vi "Main.vi"() -> ()   [LabVIEW 2016]
doc: "Use this template to create an application that executes until you click the Stop button. Unlike the Single Loop Application VI that uses polling, this VI uses the Event Structure."
uses:
  <vilib>/userdefined/High Color/IMAQdx.ctl
  <vilib>/Utility/file.llb/Write To Spreadsheet File (string).vi
  <vilib>/Utility/file.llb/Read From Spreadsheet File (string).vi
  Library_alfa.lvlib
  <vilib>/vision/driver/NI_Vision_Acquisition_Software.lvlib
  <vilib>/vision/NI_Vision_Development_Module.lvlib
panel:
  out "индикация видео":T1(plugin-control)
  in  "Media Stop Button":bool
  in  "Play Button":bool
  in  "Камера":T2
  in  "Область измерения":T3 {"Rotation" format="%.2f"; "Left" scale=0.0..1024.0; "Right" scale=0.0..1280.0}
  in  "Параметры измерения":T4={"Contrast"=40, "Filter width"=4, "Steepness"=2, "Subsampling Ratio"=5, "Show Search Area"=FALSE, "Show Search Lines"=FALSE, "Show Edges Found"=FALSE, "Show Result"=TRUE}
  in  "Рабочий цвет":u32(colorbox)
  in  "Калибровка":u32(colorbox)
  in  "Задержка":u32
  in  "Уровень бинаризации":T5={"Нижний предел"=128.0, "Верхний предел"=255.0} {"Верхний предел" format="%.2f"; "Нижний предел" format="%.2f"}
  in  "Фильтр":i32(ring)=1 items=["Red", "Green", "Blue", "Hue", "Saturation", "Luminance", "Value", "Intensity"]
  out "Индикатор камеры":bool
  in  "Blank Button":bool
  out "Индикатор камеры 2":bool
  in  "Сохранить настройки":bool
  in  "Tab Control 3":enum32{"Настройки видео", "Регулятор"}(tab)
  in  "автоматическое включение регулятора":bool caption="Автоматическое включение регулятора"
  out "Индикатор автозапуска регулятора":bool
  out "Максимальная подача (мм/мин)2":string caption="Max скорость\n(mm/min)"
  out "Boolean":bool
  in  "Регулятор":bool
  out "текущая скорость\n(mm/min)":string
  out "текущее значение\nзазора (mm)":string
  out "Задание \nзазора (mm)":string
  in  "взять зазор":bool caption="Регулятор"
  out "Марка сплава":string
  in  "Положение толкателя (mm)":dbl(slide) scale=0.0..100.0
  in  "ND HEAT BUT":bool
  in  "ND HEAT LED":bool
  out "PT 4txt":string caption="Вакуум в камере\nPT2 (torr)"
  out "PT4 2":u16(ring)
  out "NL2":u16(ring)
  in  "V5014":dbl
  out "давление 2":bool
  out "давление 1":bool
  in  "V5012_SP_He_PC2":dbl
  out "Air":bool
  in  "ПЛАЗМАТРОН В ИСХОДНОЕ":bool
  in  "Продол назад":bool
  in  "V5011_SP_He_PC2":dbl
  in  "V5010_SP_C1":dbl
  out "PT 4":string caption="Вакуум в камере\nPT2 (torr)"
  in  "PT4":dbl
  in  "M_PLasmatron":dbl
  out "V барабаны 2":dbl
  in  "Tab Control 2":enum32{"X1", "X2", "Y"}(tab)
  out "X240":bool[](array[boolean])
  out "ОП1 Х1 5":string[](array[string])
  out "X200":bool[](array[boolean])
  out "ОП1 Х1 4":string[](array[string])
  out "X140":bool[](array[boolean])
  out "ОП1 Х1 3":string[](array[string])
  out "X100":bool[](array[boolean])
  out "ОП1 Х1 2":string[](array[string])
  out "X400":bool[](array[boolean])
  out "ОП1 Х1 8":string[](array[string])
  out "X340":bool[](array[boolean])
  out "ОП1 Х1 7":string[](array[string])
  out "X300":bool[](array[boolean])
  out "ОП1 Х1 6":string[](array[string])
  out "Y120":bool[](array[boolean])
  out "ОП1 Х1 10":string[](array[string])
  out "Y60":bool[](array[boolean])
  out "ОП1 Х1 9":string[](array[string])
  out "Air 4":bool
  in  "PT3 2":dbl
  out "V вращ. бараб 2":string caption="V заготовки"
  out "LONGITUDINAL SPEED":string
  out "PLASMATRON SPEED":string
  in  "mac3":bool
  in  "Ошибка 2":i16 format="%x"
  in  "Скорость пп 2":i16
  out "Полож заг сер":bool
  out "Полож заг нач":bool caption="НАЧАЛО"
  out "Полож заг кон":bool
  out "Полож плазм кон":bool caption="Конец"
  out "Полож плазм сер":bool caption="Пром."
  out "Полож плазм  нач":bool caption="Начало"
  in  "МАКСИМАЛЬНАЯ СКОРОСТЬ ПП К":bool
  in  "v4066_cкорость подачи плазматрона":dbl
  in  "v4065_cкорость подачи":dbl
  in  "V7045_I_ist":dbl
  in  "V7045_U_ist":dbl
  in  "Действующий ток на плазматроне":string caption="Ток А"
  out "V заготовки":string
  in  "D, заготовки":i16
  in  "Закончить автораспыление":bool
  in  "Автораспыление доплавить":bool
  in  "Автораспыление начать":bool
  in  "задание тока А":string caption="Задание, А"
  in  "ПОДАЧА ЗАГОТОВКИ":bool
  in  "stop 2":bool
  in  "SP_зазор":dbl
  in  "PV_зазор":dbl
  in  "max out":dbl
  in  "out":dbl
  out "Distance зазор":sgl format="%.2f"
  out "x/y":dbl
  out "x*y":dbl
  out "16bit integer":i16
  in  "Numeric":i16
  in  "Т6":dbl
  in  "Улавливатель закрыть":bool
  in  "Улавливатель открыть":bool
  in  "Ролик прижать":bool
  in  "Ролик отжать":bool
  in  "PE3":dbl
  in  "PE2":dbl
  in  "PE1":dbl
  in  "ЗАДАНИЕ ТОКА":i16
  in  "ГС - Закрыть":bool
  in  "ГС -Открыть":bool
  out "ГС - Плазматрон":string caption="Плазматрон"
  out "ГС - Камера":string caption="Камера"
  in  "Скорость пп":i16
  in  "V барабаны задание":dbl
  in  "Выход":bool
  in  "ГС ПТ":i16
  in  "ГС камера":i16
  in  "V барабаны":dbl
  in  "Т5":dbl
  in  "Т4":dbl
  in  "Т3":dbl
  in  "Т2":dbl
  in  "Т1":dbl
  in  "Ошибка":i16
  in  "PT3":dbl
  in  "PT2":dbl
  in  "PT1":dbl
  in  "y120":i32
  in  "y60":i32
  in  "x400":i32
  in  "x340":i32
  in  "x300":i32
  in  "x240":i32
  in  "x200":i32
  in  "x140":i32
  in  "x100":i32
  in  "Tab Control":enum32{"Вакуум", "Распыление", "Осциллограмма"}(tab)
  in  "откачка стоп 2":bool
  out "Распыление":bool
  out "Вакуум":bool
  out "Газ":bool
  out "VP4":u16(ring)
  out "PD2":u16(ring)
  out "VP2":u16(ring)
  in  "Slide":dbl(slide) scale=0.0..99.0
  out "EV1":u16(ring)
  out "EV2":u16(ring)
  out "EV3.3":u16(ring)
  out "EV3.2":u16(ring)
  out "PE2":u16(ring)
  out "PE2":string caption="Вакуум в камере\nPT2 (torr)"
  out "CO1":u16(ring)
  out "CO2":u16(ring)
  out "EV3.1":u16(ring)
  out "CO3":u16(ring)
  out "P1":u16(ring)
  out "PE1":u16(ring)
  out "PE1":string caption="Вакуум в камере\nPT2 (torr)"
  out "PE3":u16(ring)
  out "PE3":string caption="Вакуум в камере\nPT2 (torr)"
  out "VP1":u16(ring)
  out "PT3":u16(ring)
  out "PT2":u16(ring)
  out "PT 2":string caption="Вакуум в камере\nPT2 (torr)"
  out "VP3":u16(ring)
  out "VP5":u16(ring)
  out "PD1":u16(ring)
  out "PT1":u16(ring)
  out "PT 1":string caption="Вакуум в камере\nPT2 (torr)"
  out "NZ1":u16(ring)
  out "NR1":u16(ring)
  out "NL1":u16(ring)
  out "PT 3":string caption="Вакуум в камере\nPT2 (torr)"
  out "SP Presure Ar PC2":string caption="SP C1 (kgf/cm^2)"
  in  "напустить аргон в ресивер":bool
  in  "mac6":bool
  out "SP Presure He PC2":string caption="SP C1 (kgf/cm^2)"
  in  "mac5":bool
  in  "напустить гелий в ресивер":bool
  out "SP Presure C1":string caption="SP C1 (kgf/cm^2)"
  in  "mac 4":bool
  in  "напустить газ в камеру":bool
  in  "forvacuum":bool
  in  "forvakuum led":bool
  in  "откачка стоп":bool
  in  "откачка стоп индик":bool
  in  "откачать рабочий вакуум":bool
  in  "mac 2":bool
  out "ИНдикатор положения полки":string
  in  "ЗУ-вверх":bool
  in  "Пауза допыления":string caption="Пауза допыления (sec)"
  out "C212":bool
  out "УГ_закрыт":bool caption="Отжат"
  out "УГ_открыт":bool caption="Прижат"
  out "ролик_отжат":bool caption="Вверху"
  out "ролик_прижат":bool caption="Внизу"
  out "max Speed":string caption="Максимальная \nСкорость (r/min)"
  out "ТЕМП КАМЕРА":string caption="T газ (C°)"
  in  "Скорость ПП 2":string caption="Скорость плазматрона\n(mm/min)"
  in  "Скорость ПП":string caption="Скорость толкателя (mm/min)"
  out "ТЕМП РОЛИК":string caption="T ролик (C°)"
  out "ПОДШ. 2.2":string caption="T4 (C°)"
  out "ПОДШ. 2.1":string caption="T3 (C°)"
  out "ПОДШ. 1.2":string caption="T2 (C°)"
  out "ПОДШ. 1.1":string caption="T1 (C°)"
  out "P плазматрон (bar)":string
  out "P камера (bar)":string
  out "I_ist":string caption="Ток (A)"
  out "U_ist":string caption="Напряжение (V)"
  out "Диаметр заг.":string caption="Диаметр (mm)"
  out "V задания":string caption="Скорость вращения (r/min)"
  out "V вращ. бараб":string caption="Частота вращения (r/min)"
  in  "ПЛАЗМАТРОН В ИСХОДНОЕ 2":bool
  out "Частота вращения":dbl(graph)
  out "Значение зазора":dbl(graph)
  out "Скорость толкателя":dbl(graph)
  out "Ток":dbl(graph)
  out "Напряжение":dbl(graph)
  out "voto plasmatron":string caption="моточасы работы\nплазматрона"
  out "текущее время":string
  in  "Arhive":bool
  # "Ролик"
  # "Улавливатель ОГ"
  # "PLASMATRON"
  # "Обработка"
  # "БАРАБАНЫ"
  # "РАСПЫЛЕНИЕ ЗАГОТОВКИ"
  # "Температура"
  # "3A3.1 X100-X137"
  # "3A3.2 X140-177"
  # "3A4 X200-X237"
  # "3A5.1 X240-X277"
  # "3A5.2 X300-X337"
  # "3A6 X340-X377"
  # "3A8 X400-X437"
  # "2A8 Y60-Y117"
  # "3A7 Y120-Y157"
  # "Положение толкателя"
  # "Положение плазматрона"
  # "Газовая система"
  # "VF1"
  # "Ar,He"
  # "PC1"
  # "PC2"
  # "Толкатель"
  # "Прижим крышки"
  # "Прижимной ролик"
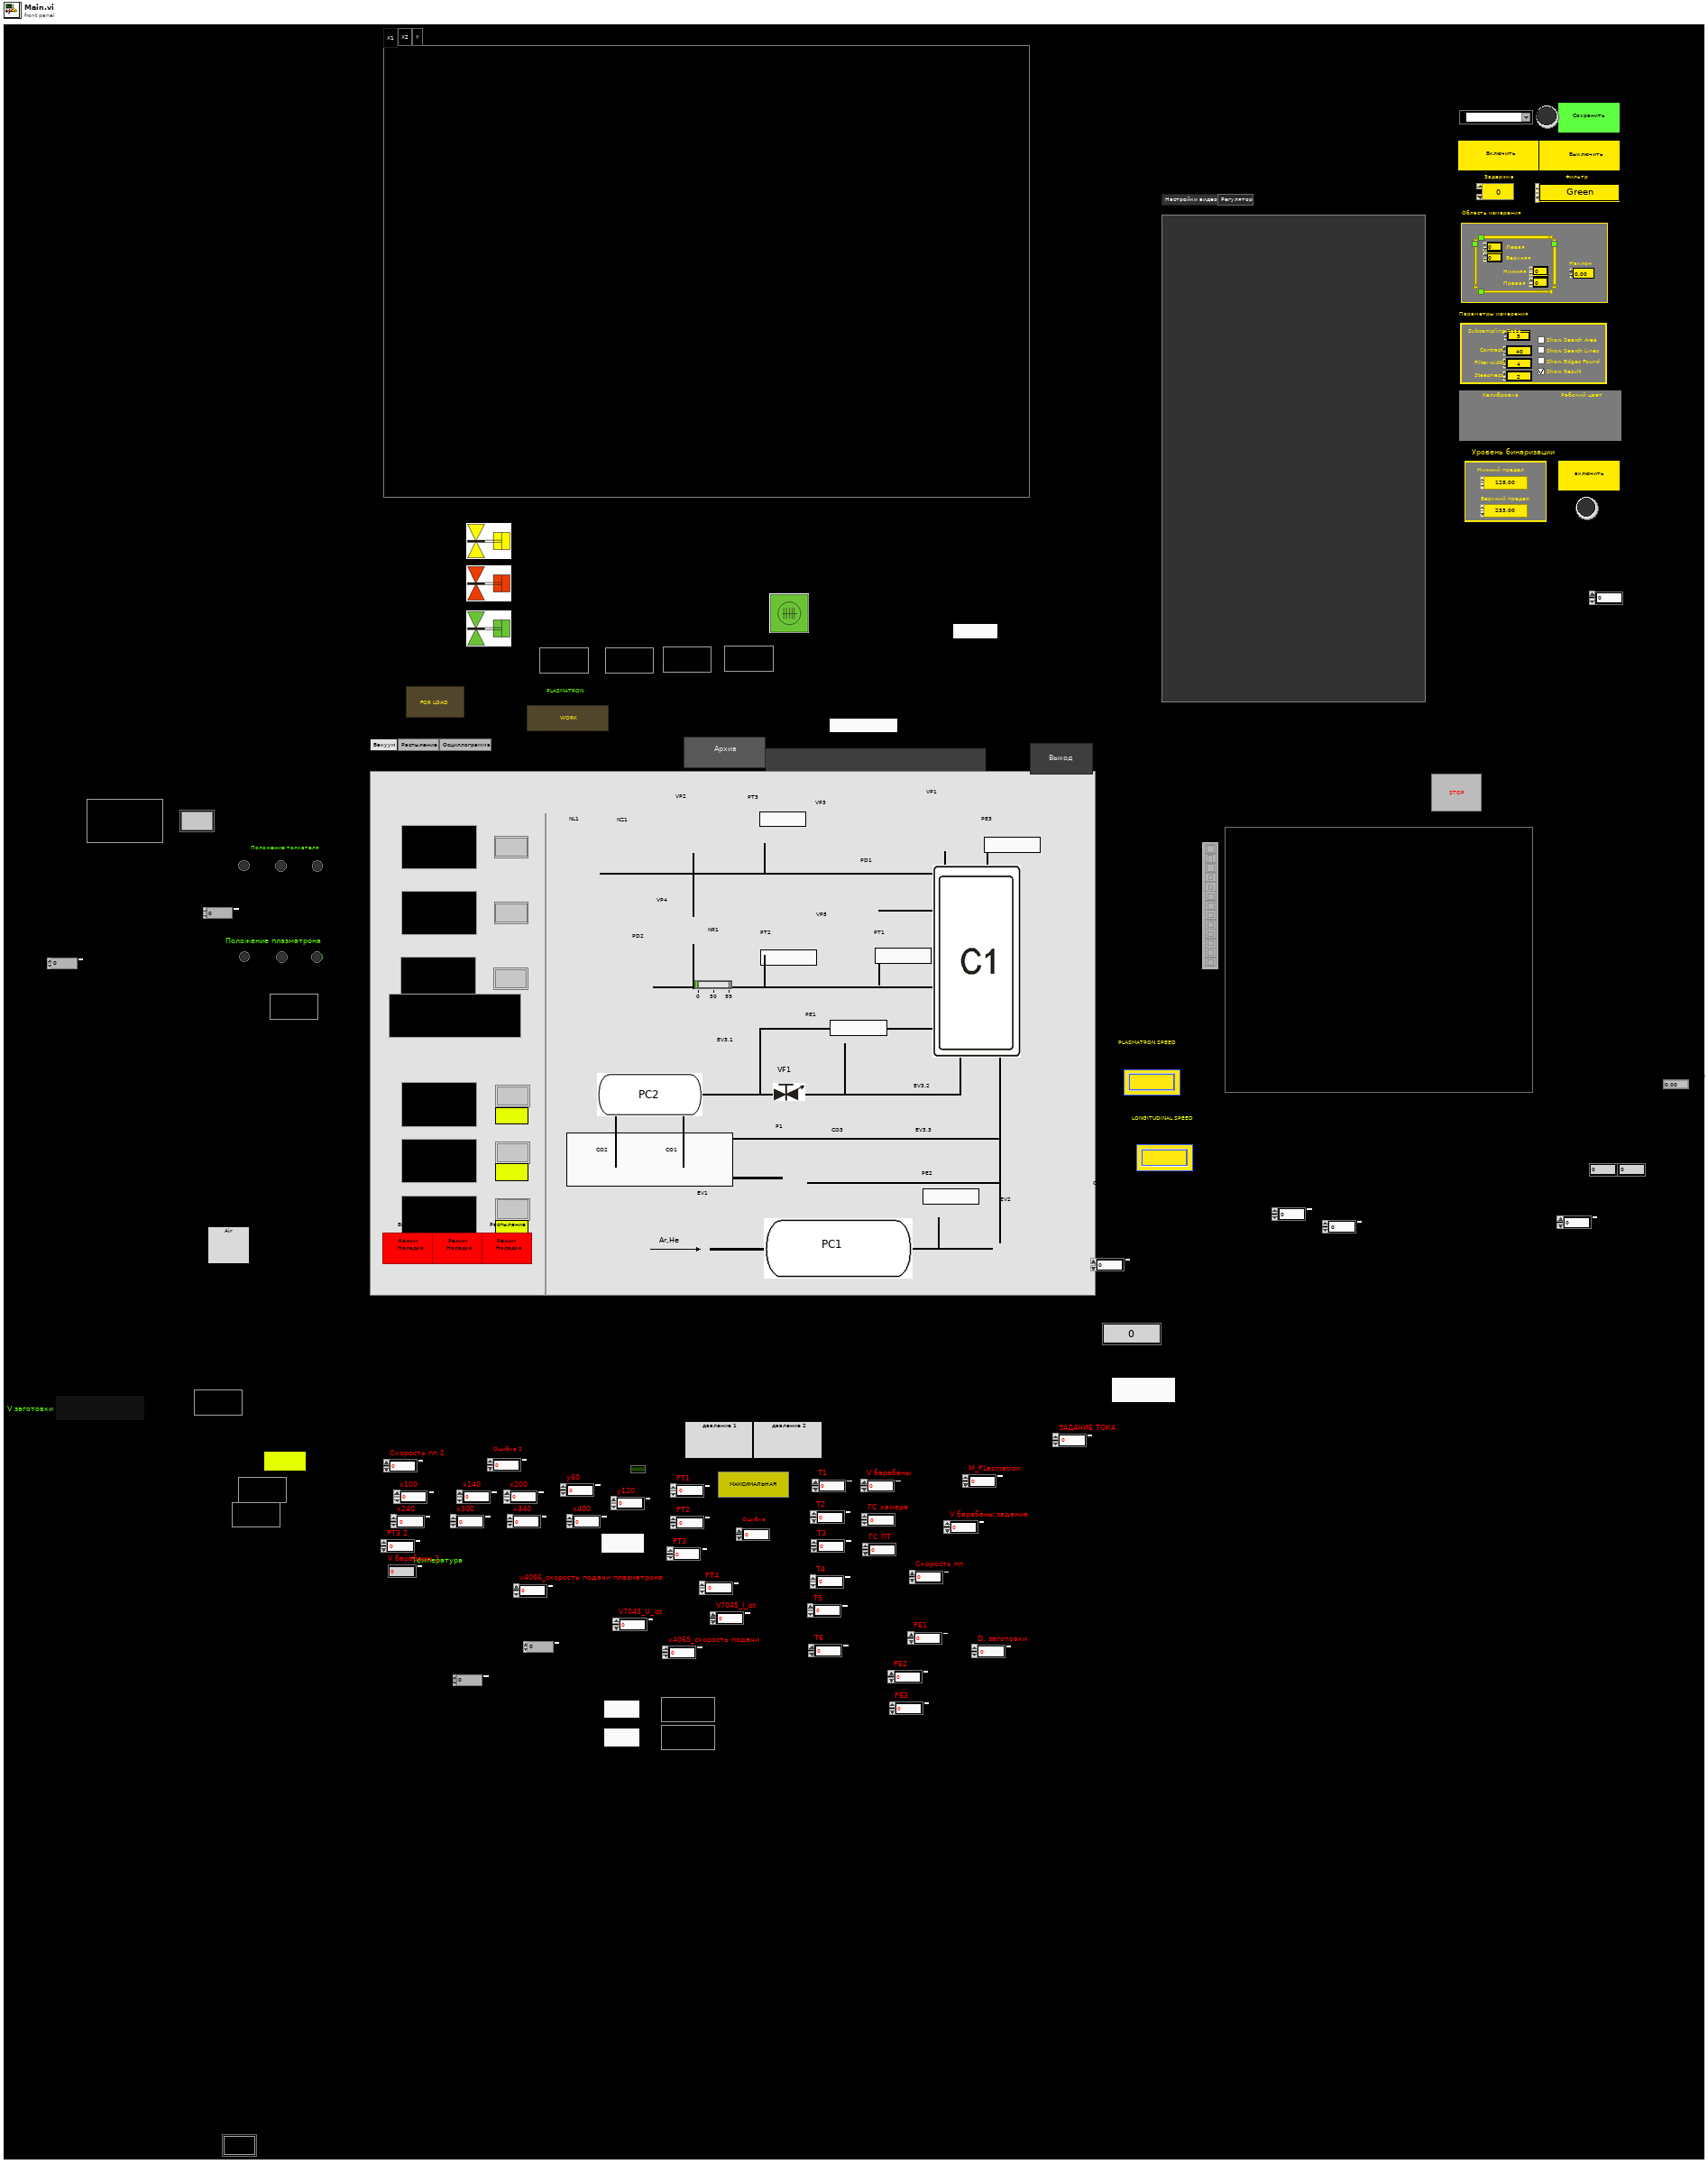
[diagram p1: front panel]
types:
  T1 = typedef "IMAQ Image.ctl" = refnum<image>
  T2 = typedef "Library_alfa.lvlib/IMAQdx.ctl" = refnum<k21>
  T3 = typedef "IMAQ Rectangle" = cluster{"Left":i32, "Top":i32, "Right":i32, "Bottom":i32, "Rotation":dbl}
  T4 = cluster{"Contrast":i32, "Filter width":i32, "Steepness":i32, "Subsampling Ratio":u32, "Show Search Area":bool, "Show Search Lines":bool, "Show Edges Found":bool, "Show Result":bool}
  T5 = cluster{"Нижний предел":sgl, "Верхний предел":sgl}
  T6 = enum16{"open", "replace", "create", "open or create", "replace or create", "replace or create with confirmation"}
  T7 = enum8{"Enabled", "Disabled", "Disabled and Grayed Out"}
  T8 = cluster{i32, i32, i32, u32, "Boolean":bool, "Boolean":bool, "Boolean":bool, "Boolean":bool}
  T9 = typedef "Image Type" = u32
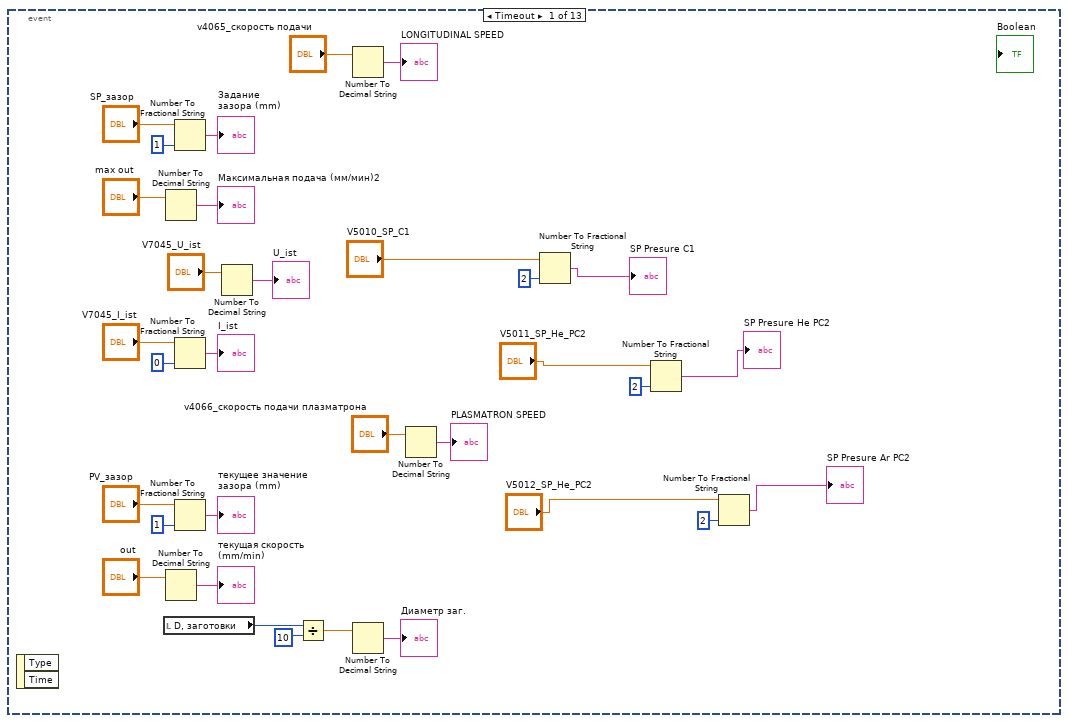
[diagram p6: hidden frame]
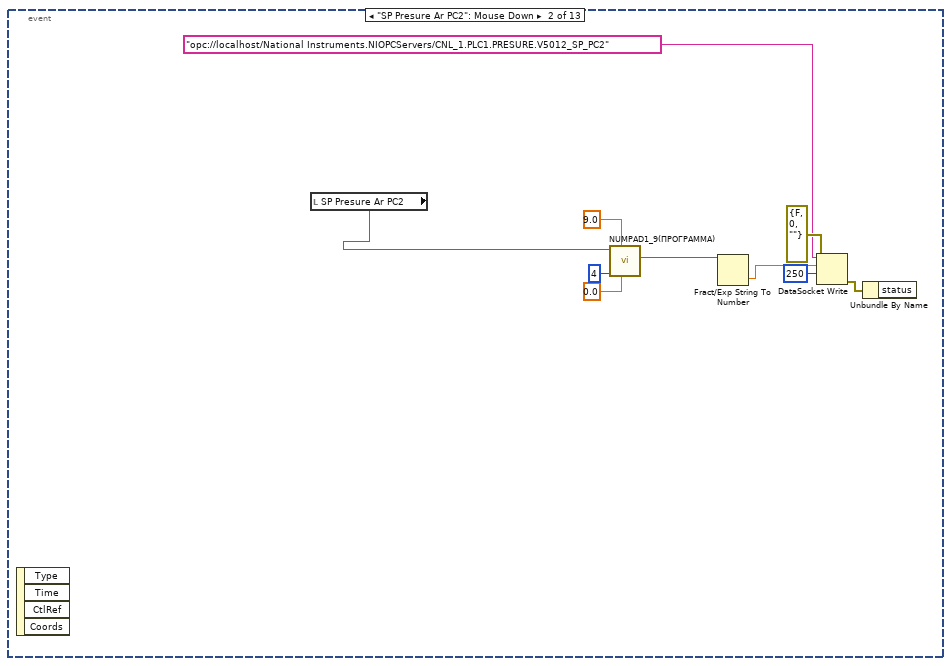
[diagram p7: hidden frame]
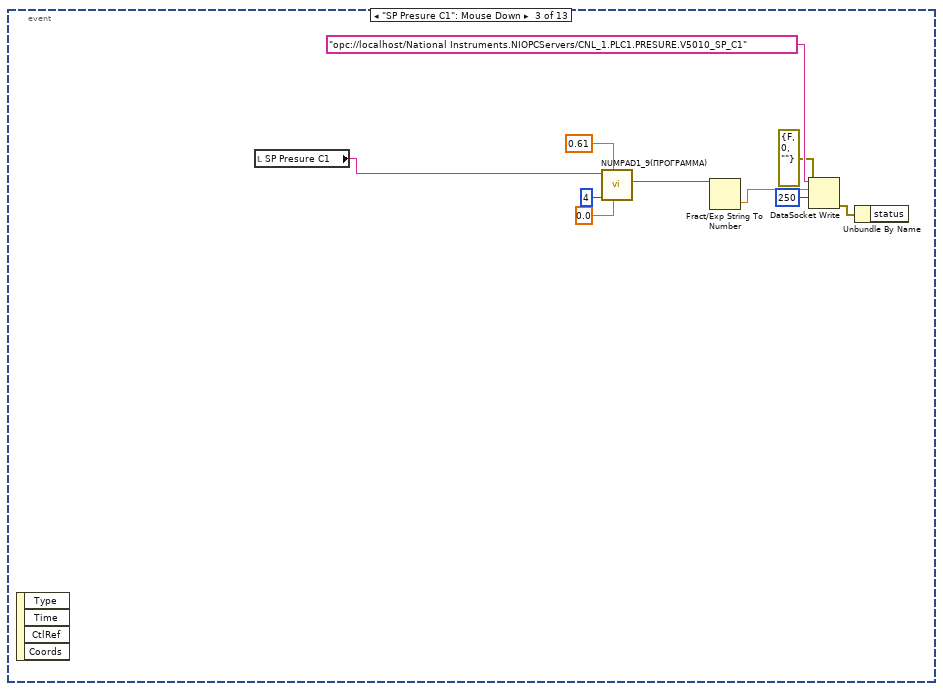
[diagram p8: hidden frame]
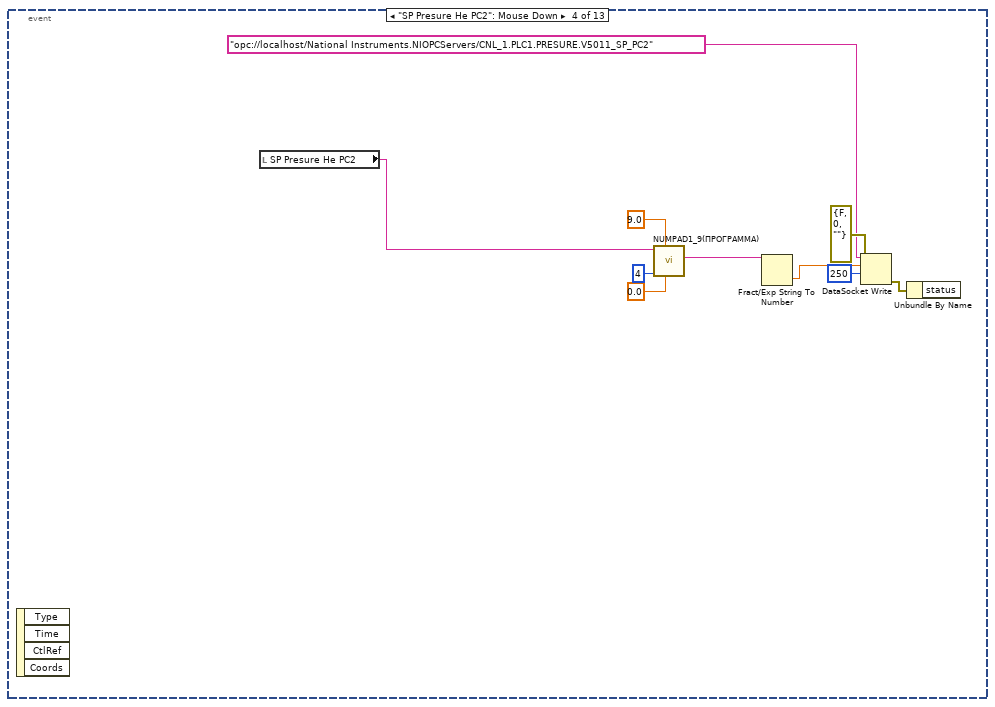
[diagram p9: hidden frame]
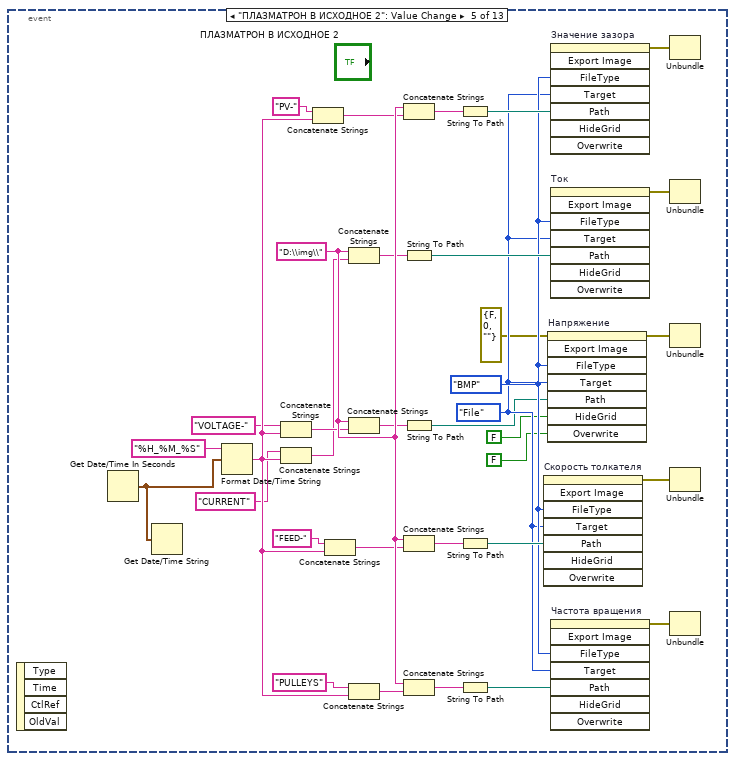
[diagram p10: hidden frame]
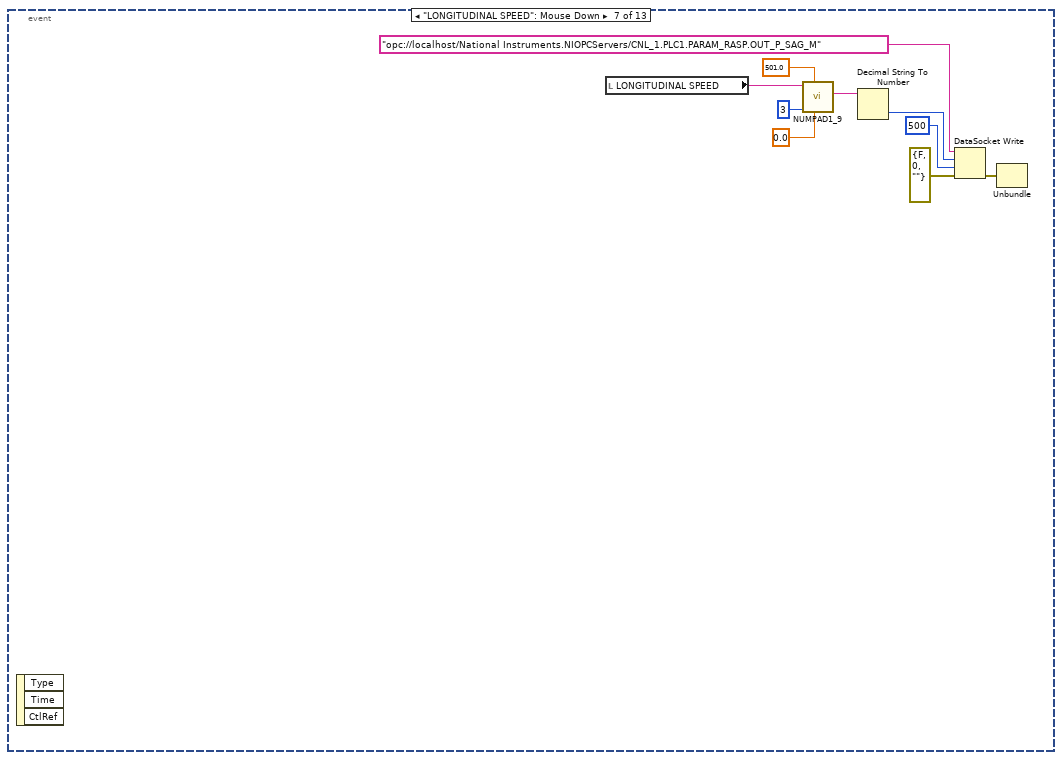
[diagram p11: hidden frame]
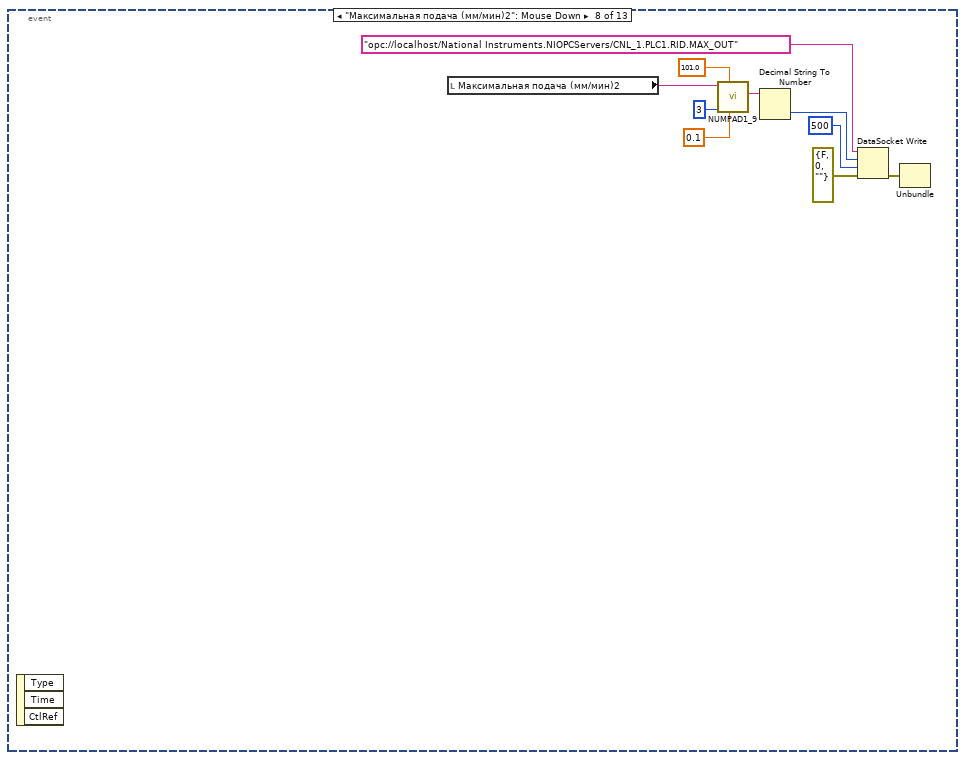
[diagram p12: hidden frame]
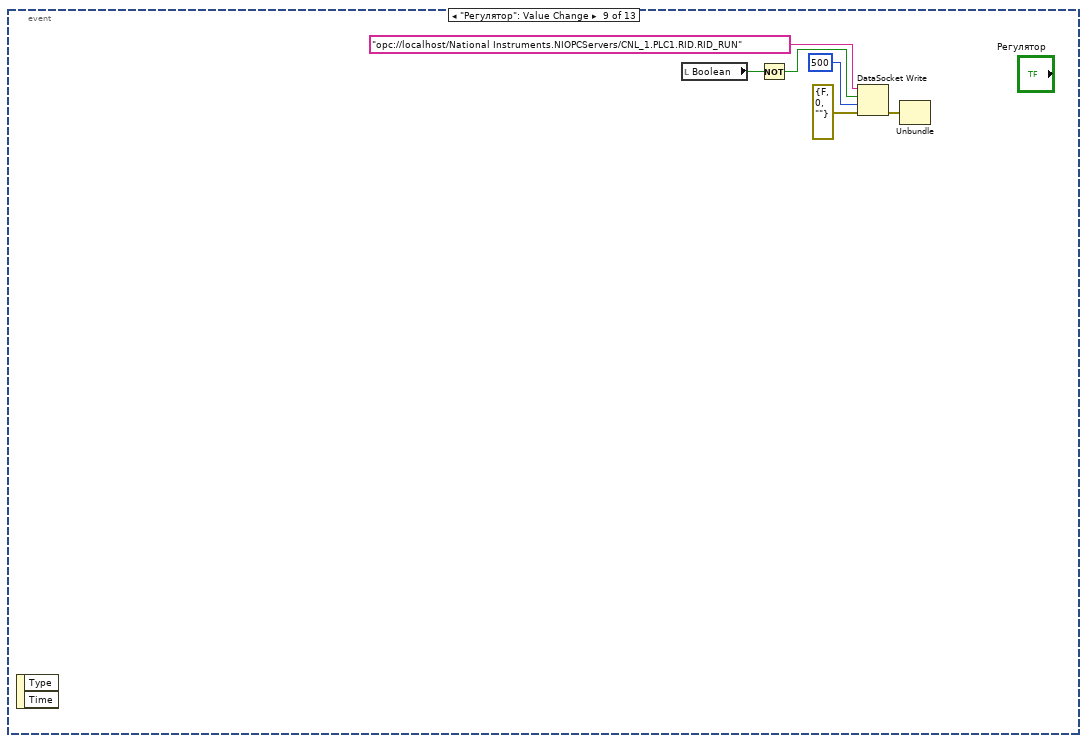
[diagram p13: hidden frame]
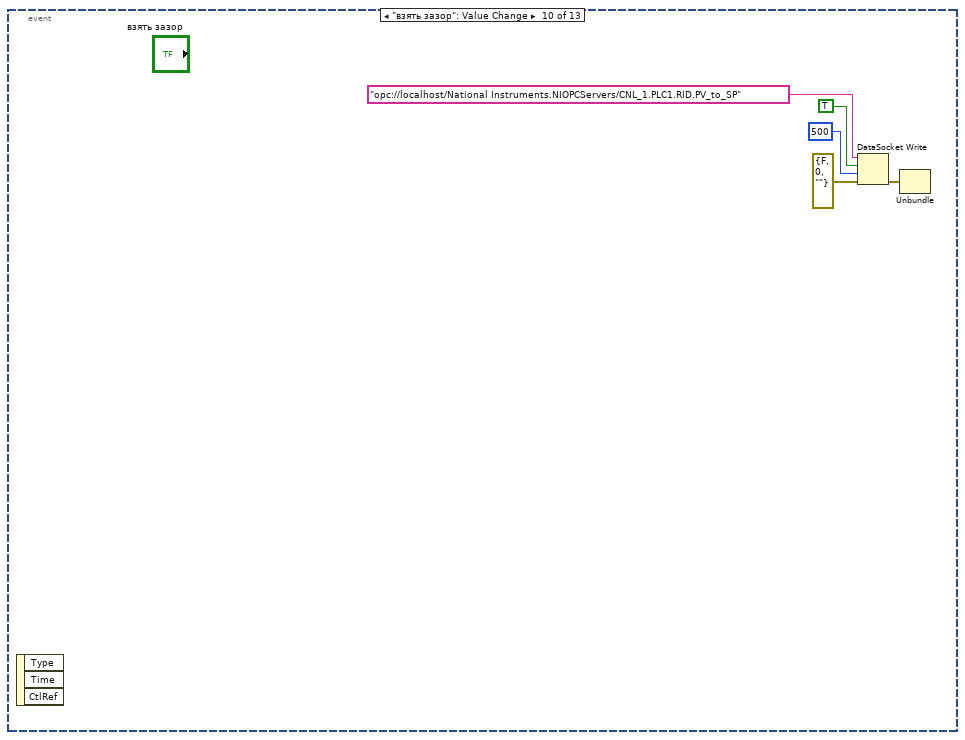
[diagram p14: hidden frame]
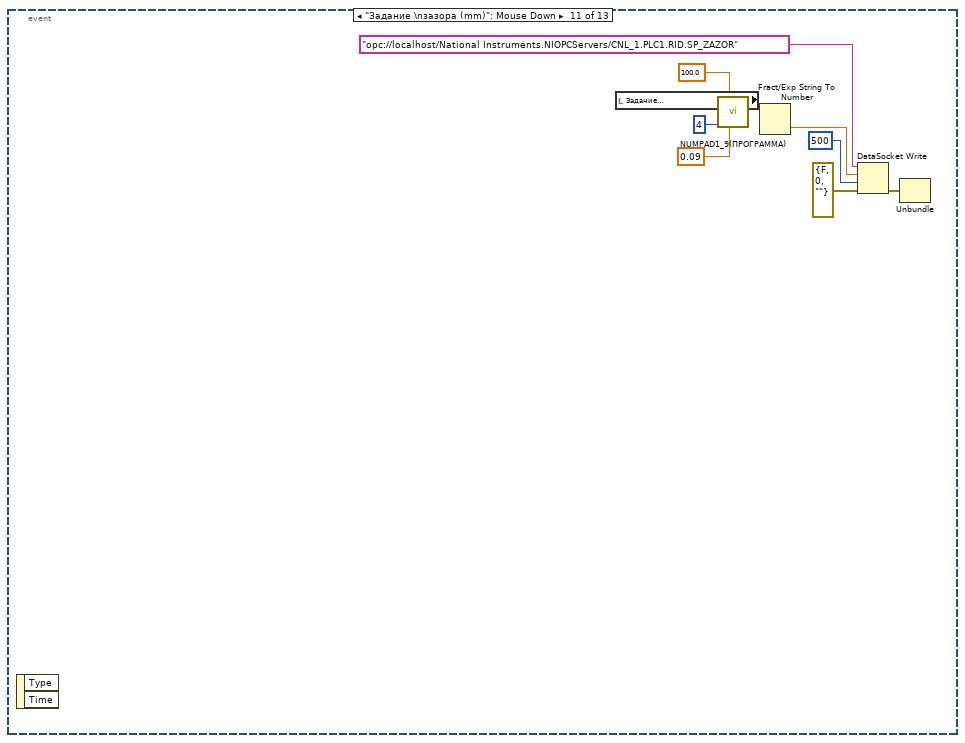
[diagram p15: hidden frame]
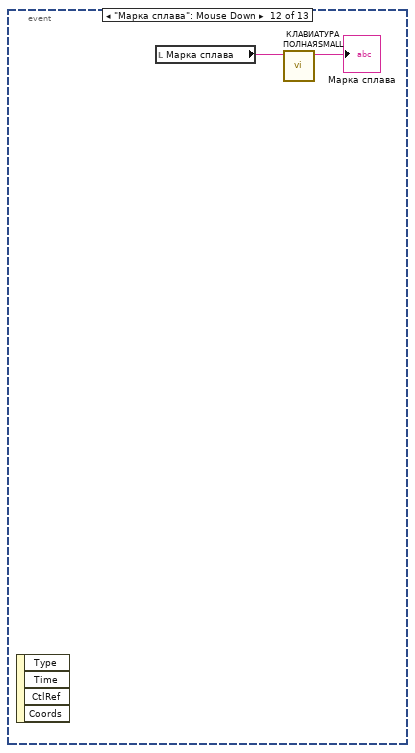
[diagram p16: hidden frame]
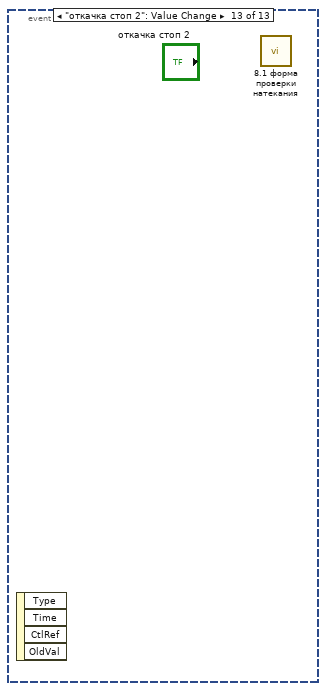
[diagram p17: hidden frame]
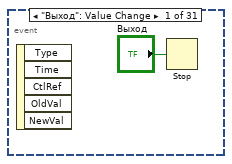
[diagram p19: hidden frame]
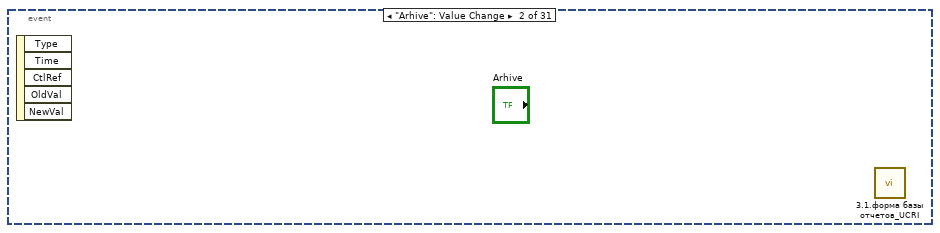
[diagram p20: hidden frame]
diagram:
  n1 = while {
    stop <- "stop 2" stop-if-true
    n2 = Wait Until Next ms Multiple(millisecond multiple=u32 250) -> ()  [unwired: 1 out]
    n3 = event shown="[5] \"PLASMATRON SPEED\": Mouse Down" {
      selector: _ -> [_ _ _ _ _ _ _ _ _ _ _ _ _]
      dyn-events: _ -> [_ _ _ _ _ _ _ _ _ _ _ _ _]
      timeout: 250 -> [_ _ _ _ _ _ _ _ _ _ _ _ _]
      event Timeout {
        n4 = event-data() -> ()  [unwired: 1 in, 2 out]
        n5 = local read "D, заготовки"() -> (w30:i16)
        n6 = Number To Decimal String(number="max out") -> (decimal integer string=→"Максимальная подача (мм/мин)2":string)  [unwired: 1 in]
        n7 = Number To Decimal String(number="out") -> (decimal integer string=→"текущая скорость\n(mm/min)":string)  [unwired: 1 in]
        n8 = Number To Fractional String(number="SP_зазор", precision (6)=i16 1) -> (F-format string=→"Задание \nзазора (mm)":string)  [unwired: 2 in]
        n9 = Number To Fractional String(number="V7045_I_ist", precision (6)=i16 0) -> (F-format string=→"I_ist":string)  [unwired: 2 in]
        n10 = Number To Fractional String(number="PV_зазор", precision (6)=i16 1) -> (F-format string=→"текущее значение\nзазора (mm)":string)  [unwired: 2 in]
        n11 = Number To Decimal String(number="V7045_U_ist") -> (decimal integer string=→"U_ist":string)  [unwired: 1 in]
        n12 = Divide(x=w30, y=i16 10) -> (x/y=w28:dbl)
        n13 = Number To Decimal String(number="v4065_cкорость подачи") -> (decimal integer string=→"LONGITUDINAL SPEED":string)  [unwired: 1 in]
        n14 = Number To Decimal String(number=w28) -> (decimal integer string=→"Диаметр заг.":string)  [unwired: 1 in]
        n15 = Number To Decimal String(number="v4066_cкорость подачи плазматрона") -> (decimal integer string=→"PLASMATRON SPEED":string)  [unwired: 1 in]
        n16 = Number To Fractional String(number="V5010_SP_C1", precision (6)=i16 2) -> (F-format string=→"SP Presure C1":string)  [unwired: 2 in]
        n17 = Number To Fractional String(number="V5011_SP_He_PC2", precision (6)=i16 2) -> (F-format string=→"SP Presure He PC2":string)  [unwired: 2 in]
        n18 = Number To Fractional String(number="V5012_SP_He_PC2", precision (6)=i16 2) -> (F-format string=→"SP Presure Ar PC2":string)  [unwired: 2 in]
      }
      event "SP Presure Ar PC2": Mouse Down {
        n19 = event-data() -> ()  [unwired: 1 in, 4 out]
        n20 = local read "SP Presure Ar PC2"() -> (w37:string)
        n21 = call "NUMPAD1_9(ПРОГРАММА).vi"("МИНИМАЛЬНОЕ ЗНАЧЕНИЕ"=0.0, "МАКСИМАЛЬНОЕ ЗНАЧЕНИЕ"=9.0, "ДЛИННА СЛОВА"=i8 4, "ТЕКУЩЕЕ ЗНАЧЕНИЕ"=w37) -> ("НОВОЕ ЗНАЧЕНИЕ"=w43:string)  [unwired: 6 in, 1 out]
        n22 = Fract/Exp String To Number(string=w43) -> (number=w42:dbl)  [unwired: 3 in, 1 out]
        n23 = DataSocket Write(8:errorcluster {"status"=FALSE, "code"=0, "source"=""} ("error in (no error)"), 9:250 ("ms timeout (0)"), 10:w42, 11:"opc://localhost/National Instruments.NIOPCServers/CNL_1.PLC1.PRESURE.V5012_SP_PC2") -> (0:w39:errorcluster)  [unwired: 2 out]
        n24 = Unbundle By Name(w39) -> ()  [unwired: 1 out]
      }
      event "SP Presure C1": Mouse Down {
        n25 = event-data() -> ()  [unwired: 1 in, 4 out]
        n26 = local read "SP Presure C1"() -> (w56:string)
        n27 = call "NUMPAD1_9(ПРОГРАММА).vi"("МИНИМАЛЬНОЕ ЗНАЧЕНИЕ"=0.0, "МАКСИМАЛЬНОЕ ЗНАЧЕНИЕ"=0.61, "ДЛИННА СЛОВА"=i8 4, "ТЕКУЩЕЕ ЗНАЧЕНИЕ"=w56) -> ("НОВОЕ ЗНАЧЕНИЕ"=w52:string)  [unwired: 6 in, 1 out]
        n28 = Fract/Exp String To Number(string=w52) -> (number=w50:dbl)  [unwired: 3 in, 1 out]
        n29 = DataSocket Write(8:errorcluster {"status"=FALSE, "code"=0, "source"=""} ("error in (no error)"), 9:250 ("ms timeout (0)"), 10:w50, 11:"opc://localhost/National Instruments.NIOPCServers/CNL_1.PLC1.PRESURE.V5010_SP_C1") -> (0:w47:errorcluster)  [unwired: 2 out]
        n30 = Unbundle By Name(w47) -> ()  [unwired: 1 out]
      }
      event "SP Presure He PC2": Mouse Down {
        n31 = event-data() -> ()  [unwired: 1 in, 4 out]
        n32 = local read "SP Presure He PC2"() -> (w58:string)
        n33 = call "NUMPAD1_9(ПРОГРАММА).vi"("МИНИМАЛЬНОЕ ЗНАЧЕНИЕ"=0.0, "МАКСИМАЛЬНОЕ ЗНАЧЕНИЕ"=9.0, "ДЛИННА СЛОВА"=i8 4, "ТЕКУЩЕЕ ЗНАЧЕНИЕ"=w58) -> ("НОВОЕ ЗНАЧЕНИЕ"=w63:string)  [unwired: 6 in, 1 out]
        n34 = Fract/Exp String To Number(string=w63) -> (number=w62:dbl)  [unwired: 3 in, 1 out]
        n35 = DataSocket Write(8:errorcluster {"status"=FALSE, "code"=0, "source"=""} ("error in (no error)"), 9:250 ("ms timeout (0)"), 10:w62, 11:"opc://localhost/National Instruments.NIOPCServers/CNL_1.PLC1.PRESURE.V5011_SP_PC2") -> (0:w59:errorcluster)  [unwired: 2 out]
        n36 = Unbundle By Name(w59) -> ()  [unwired: 1 out]
      }
      event "ПЛАЗМАТРОН В ИСХОДНОЕ 2": Value Change {
        w100 = "D:\\img\\"
        w89 = enum32{"File", "Clipboard"}."File" ("Target")
        w90 = enum32{"BMP", "EPS", "EMF", "PICT"}."BMP" ("File Type")
        n37 = event-data() -> ()  [unwired: 1 in, 4 out]
        n38 = Get Date/Time In Seconds() -> (seconds since 1Jan1904=w79:timestamp)
        n39 = Get Date/Time String(seconds (now)=w79) -> ()  [unwired: 2 in, 2 out]
        n40 = Format Date/Time String(time format string (%c)="%H_%M_%S", seconds (now)=w79) -> (date/time string=w75:string)  [unwired: 1 in]
        n41 = Concatenate Strings("VOLTAGE-", w75) -> (w73:string)
        n42 = Concatenate Strings("CURRENT", w75) -> (w71:string)
        n43 = Concatenate Strings("PV-", w75) -> (w77:string)
        n44 = Concatenate Strings("FEED-", w75) -> (w67:string)
        n45 = Concatenate Strings(w100, w71) -> (w97:string)
        n46 = Concatenate Strings(w100, w73) -> (w99:string)
        n47 = Concatenate Strings("PULLEYS", w75) -> (w69:string)
        n48 = Concatenate Strings(w100, w77) -> (w98:string)
        n49 = String To Path(string=w97) -> (path=w93:path)
        n50 = String To Path(string=w99) -> (path=w80:path)
        n51 = Concatenate Strings(w100, w67) -> (w95:string)
        n52 = Concatenate Strings(w100, w69) -> (w96:string)
        n53 = String To Path(string=w98) -> (path=w94:path)
        n54 = String To Path(string=w95) -> (path=w91:path)
        n55 = String To Path(string=w96) -> (path=w92:path)
        n56 = invoke on="Скорость толкателя" class="WFChart (strict)" method="Export Image"("FileType"=w90, "Target"=w89, "Path"=w91) -> (error out=w84:errorcluster)  [unwired: 5 in, 7 out]
        n57 = invoke on="Напряжение" class="WFChart (strict)" method="Export Image"(error in=errorcluster {"status"=FALSE, "code"=0, "source"=""} ("error in (no error)"), "FileType"=w90, "Target"=w89, "Path"=w80, "HideGrid"=FALSE ("Hide Grid"), "Overwrite"=FALSE ("Always Overwrite")) -> (error out=w88:errorcluster)  [unwired: 2 in, 7 out]
        n58 = invoke on="Значение зазора" class="WFChart (strict)" method="Export Image"("FileType"=w90, "Target"=w89, "Path"=w94) -> (error out=w87:errorcluster)  [unwired: 5 in, 7 out]
        n59 = invoke on="Ток" class="WFChart (strict)" method="Export Image"("FileType"=w90, "Target"=w89, "Path"=w93) -> (error out=w86:errorcluster)  [unwired: 5 in, 7 out]
        n60 = invoke on="Частота вращения" class="WFChart (strict)" method="Export Image"("FileType"=w90, "Target"=w89, "Path"=w92) -> (error out=w85:errorcluster)  [unwired: 5 in, 7 out]
        n61 = Unbundle(w87) -> ()  [unwired: 3 out]
        n62 = Unbundle(w86) -> ()  [unwired: 3 out]
        n63 = Unbundle(w88) -> ()  [unwired: 3 out]
        n64 = Unbundle(w84) -> ()  [unwired: 3 out]
        n65 = Unbundle(w85) -> ()  [unwired: 3 out]
      }
      event "PLASMATRON SPEED": Mouse Down {
        n66 = event-data() -> ()  [unwired: 1 in, 3 out]
        n67 = local read "PLASMATRON SPEED"() -> (w101:string)
        n68 = call "NUMPAD1_9.vi"("МИНИМАЛЬНОЕ ЗНАЧЕНИЕ"=0.0, "МАКСИМАЛЬНОЕ ЗНАЧЕНИЕ"=501.0, "ДЛИННА СЛОВА"=i8 3, "ТЕКУЩЕЕ ЗНАЧЕНИЕ"=w101) -> ("НОВОЕ ЗНАЧЕНИЕ"=w103:string)  [unwired: 7 in]
        n69 = Decimal String To Number(string=w103) -> (number=w106:i32)  [unwired: 2 in, 1 out]
        n70 = DataSocket Write(8:errorcluster {"status"=FALSE, "code"=0, "source"=""} ("error in (no error)"), 9:500 ("ms timeout (0)"), 10:w106, 11:"opc://localhost/National Instruments.NIOPCServers/CNL_1.PLC1.PARAM_RASP.SP_PR_PLAZM") -> (0:w109:errorcluster)  [unwired: 2 out]
        n71 = Unbundle(w109) -> ()  [unwired: 3 out]
      }
      event "LONGITUDINAL SPEED": Mouse Down {
        n72 = event-data() -> ()  [unwired: 1 in, 3 out]
        n73 = local read "LONGITUDINAL SPEED"() -> (w114:string)
        n74 = call "NUMPAD1_9.vi"("МИНИМАЛЬНОЕ ЗНАЧЕНИЕ"=0.0, "МАКСИМАЛЬНОЕ ЗНАЧЕНИЕ"=501.0, "ДЛИННА СЛОВА"=i8 3, "ТЕКУЩЕЕ ЗНАЧЕНИЕ"=w114) -> ("НОВОЕ ЗНАЧЕНИЕ"=w112:string)  [unwired: 7 in]
        n75 = Decimal String To Number(string=w112) -> (number=w116:i32)  [unwired: 2 in, 1 out]
        n76 = DataSocket Write(8:errorcluster {"status"=FALSE, "code"=0, "source"=""} ("error in (no error)"), 9:500 ("ms timeout (0)"), 10:w116, 11:"opc://localhost/National Instruments.NIOPCServers/CNL_1.PLC1.PARAM_RASP.OUT_P_SAG_M") -> (0:w119:errorcluster)  [unwired: 2 out]
        n77 = Unbundle(w119) -> ()  [unwired: 3 out]
      }
      event "Максимальная подача (мм/мин)2": Mouse Down {
        n78 = event-data() -> ()  [unwired: 1 in, 3 out]
        n79 = local read "Максимальная подача (мм/мин)2"() -> (w121:string)
        n80 = call "NUMPAD1_9.vi"("МИНИМАЛЬНОЕ ЗНАЧЕНИЕ"=0.1, "МАКСИМАЛЬНОЕ ЗНАЧЕНИЕ"=101.0, "ДЛИННА СЛОВА"=i8 3, "ТЕКУЩЕЕ ЗНАЧЕНИЕ"=w121) -> ("НОВОЕ ЗНАЧЕНИЕ"=w123:string)  [unwired: 7 in]
        n81 = Decimal String To Number(string=w123) -> (number=w122:i32)  [unwired: 2 in, 1 out]
        n82 = DataSocket Write(8:errorcluster {"status"=FALSE, "code"=0, "source"=""} ("error in (no error)"), 9:500 ("ms timeout (0)"), 10:w122, 11:"opc://localhost/National Instruments.NIOPCServers/CNL_1.PLC1.RID.MAX_OUT") -> (0:w129:errorcluster)  [unwired: 2 out]
        n83 = Unbundle(w129) -> ()  [unwired: 3 out]
      }
      event "Регулятор": Value Change {
        n84 = event-data() -> ()  [unwired: 1 in, 2 out]
        n85 = local read "Boolean"() -> (w132:bool)
        n86 = Not(x=w132) -> (.not. x?=w131:bool)
        n87 = DataSocket Write(8:errorcluster {"status"=FALSE, "code"=0, "source"=""} ("error in (no error)"), 9:500 ("ms timeout (0)"), 10:w131, 11:"opc://localhost/National Instruments.NIOPCServers/CNL_1.PLC1.RID.RID_RUN") -> (0:w135:errorcluster)  [unwired: 2 out]
        n88 = Unbundle(w135) -> ()  [unwired: 3 out]
      }
      event "взять зазор": Value Change {
        n89 = event-data() -> ()  [unwired: 1 in, 3 out]
        n90 = DataSocket Write(8:errorcluster {"status"=FALSE, "code"=0, "source"=""} ("error in (no error)"), 9:500 ("ms timeout (0)"), 10:TRUE, 11:"opc://localhost/National Instruments.NIOPCServers/CNL_1.PLC1.RID.PV_to_SP") -> (0:w139:errorcluster)  [unwired: 2 out]
        n91 = Unbundle(w139) -> ()  [unwired: 3 out]
      }
      event "Задание \nзазора (mm)": Mouse Down {
        n92 = event-data() -> ()  [unwired: 1 in, 2 out]
        n93 = local read "Задание \nзазора (mm)"() -> (w144:string)
        n94 = call "NUMPAD1_9(ПРОГРАММА).vi"("МИНИМАЛЬНОЕ ЗНАЧЕНИЕ"=0.09, "МАКСИМАЛЬНОЕ ЗНАЧЕНИЕ"=100.0, "ДЛИННА СЛОВА"=i8 4, "ТЕКУЩЕЕ ЗНАЧЕНИЕ"=w144) -> ("НОВОЕ ЗНАЧЕНИЕ"=w145:string)  [unwired: 6 in, 1 out]
        n95 = Fract/Exp String To Number(string=w145) -> (number=w142:dbl)  [unwired: 3 in, 1 out]
        n96 = DataSocket Write(8:errorcluster {"status"=FALSE, "code"=0, "source"=""} ("error in (no error)"), 9:500 ("ms timeout (0)"), 10:w142, 11:"opc://localhost/National Instruments.NIOPCServers/CNL_1.PLC1.RID.SP_ZAZOR") -> (0:w150:errorcluster)  [unwired: 2 out]
        n97 = Unbundle(w150) -> ()  [unwired: 3 out]
      }
      event "Марка сплава": Mouse Down {
        n98 = event-data() -> ()  [unwired: 1 in, 4 out]
        n99 = local read "Марка сплава"() -> (w152:string)
        n100 = call "КЛАВИАТУРА ПОЛНАЯSMALL.vi"("ВХОД СТАРОЕ"=w152) -> ("ВЫХОД РЕЗУЛЬТАТ"=→"Марка сплава":string)  [unwired: 10 in]
      }
      event "откачка стоп 2": Value Change {
        n101 = event-data() -> ()  [unwired: 1 in, 4 out]
        n102 = call "8.1 форма проверки натекания.vi"() -> ()  [unwired: 1 in]
      }
    }
  }
  n103 = flat-sequence {
    tunnel: [w155] -> w1
    tunnel: w1 -> [w213]
    frame #0 {
      # "Экран наладки - подписи"
      n104 = local write "Tab Control 3"(enum32{"Настройки видео", "Регулятор"}."Регулятор" ("Tab Control 3")) -> ()
      n105 = Number To Decimal String(number="ГС ПТ") -> (decimal integer string=→"ГС - Плазматрон":string)  [unwired: 1 in]
      n106 = Number To Decimal String(number="ГС камера") -> (decimal integer string=→"ГС - Камера":string)  [unwired: 1 in]
      n107 = call "путь для общего отчета.vi"() -> ("path_out 2"=w161:string)  [unwired: 11 in]
      n108 = Spreadsheet String To Array(delimiter (Tab)="\n", format string="", spreadsheet string="ОТК открыта\nОТК  закрыта\nОТК закрыть\nОТК  открыть\nПУ вправо\nПУ влево\nПУ крут влево\nПУ крут вправо\nРГ продувка\nРГ окисленные\nРГ окисленныек\nРГ кондиционк\nРГ кондицион\nРГ проба\nРГ пробак\nРГ кондиционкк\nРГ продувка\nРГ окисленные\nЗУ вверх\nЗУ вниз\nЗУ вверху\nЗУ 1 полка\nЗУ 2 полка\nЗУ 3 полка\nЗУ 4 полка\nЗУ 5 полка\nЗУ 6 полка\nЗУ 7 полка\nЗУ 8 полка\nЗУ 9 полка\nЗУ 10 полка\nУровень 1 < N", array type (2D Dbl)=string[] [] ("ОП1 Х1")) -> (array=→"ОП1 Х1 6":string[])
      n109 = Spreadsheet String To Array(delimiter (Tab)="\n", format string="", spreadsheet string="Питание 24В вкл\nПЛК / Наладка\nNL включен\nNL включить\nNL выключить\nNZ включен\nNZ включить\nNZ выключить\nNB включен\nNB включить\nNB выключить\nVP1 закрыт\nVP1 открыт\nVP1 открыть\nVP1 закрыть\nempty\nVP2 закрыт\nVP2 открыт\nVP2 открыть\nVP2 закрыть\nVP3 закрыт\nVP3 открыт\nVP3 открыть\nVP3 закрыть\nVP4 закрыт\nVP4 открыт\nVP4 открыть\nVP4 закрыть\nVP5 закрыт\nVP5 открыт\nVP5 открыть\nVP5 закрыть", array type (2D Dbl)=string[] [] ("ОП1 Х1")) -> (array=→"ОП1 Х1 2":string[])
      n110 = Spreadsheet String To Array(delimiter (Tab)="\n", format string="", spreadsheet string="Дверь откат. Отжата\nДверь откат. Прижата\nДверь откат. Отжать\nДверь откат. Прижать\nУровень 3<N\nempty\nКлапан КЭ 1 открыть\nКлапан КЭ 1 закрыть\nКлапан КЭ 2 открыть\nКлапан КЭ 3 закрыть\nКлапан КЭ 3 открыть\nКлапан КЭ 3 закрыть\nКлапан КЭ 4 открыть\nКлапан КЭ 4 закрыть\nempty\nempty\nempty\nempty\nempty\nempty\nempty\nempty\nempty\nempty\nempty\nempty\nempty\nempty\nempty\nempty\nempty\nempty", array type (2D Dbl)=string[] [] ("ОП1 Х1")) -> (array=→"ОП1 Х1 8":string[])
      n111 = Spreadsheet String To Array(delimiter (Tab)="\n", format string="", spreadsheet string="Компр 3 вкл к\nВоздуходувка вкл\nВоздуходув вкл к\nБак3 нагр вкл к\nempty\nБак3 нагрев вкл\nempty\nempty\nempty\nempty\nempty\nempty\nempty\nempty\nempty\nempty\nempty\nempty\nempty\nempty\nempty\nempty\nempty\nempty\nempty\nempty\nempty\nempty\nempty\nempty\nempty\nempty", array type (2D Dbl)=string[] [] ("ОП1 Х1")) -> (array=→"ОП1 Х1 7":string[])
      n112 = Spreadsheet String To Array(delimiter (Tab)="\n", format string="", spreadsheet string="NL включить в\nNZ включить в\nNB включить в\nVP1 открыть в\nVP2 открыть в\nVP3 открыть в\nVP4 открыть в\nVP5 открыть в\nVP6 открыть в\nБак 3 нагрев вкл\nКлапан КЭ 1 открыть\nКлапан КЭ 2 открыть\nКлапан КЭ 3 открыть\nЗаготовка на барабан\nПрижимной ролик вверх\nПрижимной ролик вниз\nУл. огарков закрыть\nУл. огарков открыть\nПрод. Привод назад\nПрод. Привод вперед\nПлазматрон от заготовки\nПлазматрон к заготовке\nБарабаны пуск\nКлапан КЭ4 открыть\nempty\nempty\nempty\nempty\nempty\nempty\nempty\nempty", array type (2D Dbl)=string[] [] ("ОП1 Х1")) -> (array=→"ОП1 Х1 9":string[])
      n113 = Spreadsheet String To Array(delimiter (Tab)="\n", format string="", spreadsheet string="Крышка загр. Прижата\nКрышка загр. Отжата\nКрышка загр. Отжать\nКрышка загр. Прижать\nКрышка загр. Открыта\nКрышка загр. Закрыта\nКрышка загр. Закрыть\nКрышка загр. Открыть\nЗатвор гран.пров. Закрыт\nЗатвор гран.пров. Открыт\nЗатвор гран.пров. Открыть\nЗатвор гран.пров. Закрыть\nЗатвор гран.пров. Закрыт   2\nЗатвор гран.пров. Открыт   2\nЗатвор гран.пров. Закрыть  2\nЗатвор гран.пров. Открыть  2\nP возд. < N\nP газа < N\nP нк1 <N\nP нк2 <N\nСброс ошибки\nНасос 1 вкл\nНасос 2 вкл\nНасос 3 вкл\nНасос 1 вклк\nНасос 2 вклк\nНасос 3 вклк\nКомпрессор 1 вкл\nКомпрессор 2 вкл\nКомпрессор 3 вкл\nКомпр 1 вкл к\nКомпр 2 вкл к", array type (2D Dbl)=string[] [] ("ОП1 Х1")) -> (array=→"ОП1 Х1 5":string[])
      n114 = Concatenate Strings(w161, "proc.txt") -> (w163:string)
      n115 = Spreadsheet String To Array(delimiter (Tab)="\n", format string="", spreadsheet string="Закрыть дверь ОТК\nОткрыть дверь ОТК\nПересыпное вправо\nПересыпное влево\nРГ окисленные\nРГ кондицион\nРГ кондицион\nРГ проба\nРГ окисленные\nРГ продувка\nЗУ вниз\nЗУ вниз\nКрышка загр. Отжать\nКрышка загр. Прижать\nКрышка загр. Закрыть\nКрышка загр. Открыть\nempty\nЗатвор гранулопровода открыть  2\nОшибка\nАвария\nНасос1 вкл\nНасос 2 вкл\nНасос 3 вкл\nКомпрессор 1 вкл\nКомпрессор 2 вкл\nКомпрессор 3 вкл\nВоздуходувка вкл\nАвария\nempty\nЗатвор гранулопровода открыть\nДверь откат отжать\nДверь откат прижать", array type (2D Dbl)=string[] [] ("ОП1 Х1")) -> (array=→"ОП1 Х1 10":string[])
      n116 = String To Path(string=w163) -> (path=w159:path)
      n117 = Spreadsheet String To Array(delimiter (Tab)="\n", format string="", spreadsheet string="VP6 закрыт\nVP6 открыт\nVP6 открыть\nVP6 закрыть\nPT1\nPT2\nPT3\nempty\nКамераЗагруз 0   (PD1)\nКамераЗагруз -1   (PD1)\nНасос NB 0 (PD2)\nНасос NB -1 (PD2)\nempty\nempty\nempty\nempty\nИст вкл(ДУГА)\nКонтроллер управление источником\nАвария привода\nПривод готов (заготовки)\nПривод включен(заготовки)\nЗаготовка на барабан(датчик)\nЗаготовка на барабан(от выхода Y)\nПрижимной ролик вверху\nприжимной ролик внизу\nПР вниз\nПР вверх\nУл. огарков открыт\nУл. огарков закрыт\nУл. огарков закрыть\nУл. огарков открыть\nempty", array type (2D Dbl)=string[] [] ("ОП1 Х1")) -> (array=→"ОП1 Х1 3":string[])
      n118 = Open/Create/Replace File(file path (use dialog)=w159, operation (0:open)=T6."open or create") -> (refnum out=w156:refnum<file>, error out=w157:errorcluster)  [unwired: 4 in, 1 out]
      n119 = Spreadsheet String To Array(delimiter (Tab)="\n", format string="", spreadsheet string="Частотный питание включено(плазматрон)\nПродольная подача пит. Включено\nБарабаны питание включено\nПрод.привод впередк\nПрод. Привод назадк\nПрод привод дост. F\nПрод.привод готов\nпрод. Привод авария\nпрод.привод впередд\nпрод.привод назадд\nПлазматрон к заготовкек\nПлазматрон от заготовки\nдост f   плазматрон\nготов (плазматрон)\nавария плазматрон\nПлазматрон к заготовкед\nПлазматрон от заготовки\nПлазматрон к заготовке рабочее положение\nплазматро от заготовки рабочее положение\nБарабаны пуск\nБарабаны стоп\nПривод готов барабан 1\nавария привода барабана 1\nпитание включено барабаны\nбарабаны включены\nавария привода барабана 2\nпривод готов барабан 2\nПеремещение плазматрона пит. Включено\nempty\nПрижимной ролик вверху\nПрижимной ролик внизу\nempty", array type (2D Dbl)=string[] [] ("ОП1 Х1")) -> (array=→"ОП1 Х1 4":string[])
      n120 = Close File(refnum=w156, error in=w157) -> (path=w155:path, error out=w160:errorcluster)
      n121 = Unbundle(w160) -> ()  [unwired: 3 out]
    }
    frame #1 {
      n122 = while {
        stop <- FALSE stop-if-true
        w584 = i16 1 ("precision (6)")
        # "Вакуумная"
        n123 = local read "Y120"() -> (w722:bool[])
        n124 = local read "X200"() -> (w784:bool[])
        n125 = local read "X240"() -> (w768:bool[])
        n126 = local read "X100"() -> (w600:bool[])
        n127 = local read "X300"() -> (w743:bool[])
        n128 = local read "X340"() -> (w729:bool[])
        n129 = local read "X140"() -> (w803:bool[])
        n130 = local read "X400"() -> (w658:bool[])
        n131 = local read "Y60"() -> (w723:bool[])
        n132 = local read "out"() -> (→"Скорость толкателя":dbl)
        n133 = Get Date/Time In Seconds() -> (seconds since 1Jan1904=w667:timestamp)
        n134 = Wait Until Next ms Multiple(millisecond multiple=u32 500) -> ()  [unwired: 1 out]
        n135 = local read "V7045_U_ist"() -> (→"Напряжение":dbl)
        n136 = local read "V7045_I_ist"() -> (→"Ток":dbl)
        n137 = local read "PV_зазор"() -> (→"Значение зазора":dbl)
        n138 = local read "X140"() -> (w634:bool[])
        n139 = call "Метакон.vi"("Vak_in"="PT2") -> ("Vak_out_txt"=→"PT 2":string)  [unwired: 9 in, 1 out]
        n140 = call "Метакон.vi"("Vak_in"="PT3") -> ("Vak_out_txt"=→"PT 3":string)  [unwired: 9 in, 1 out]
        n141 = call "Метакон.vi"("Vak_in"="PT1") -> ("Vak_out_txt"=→"PT 1":string)  [unwired: 9 in, 1 out]
        n142 = Format Date/Time String(seconds (now)=w667) -> (date/time string=→"текущее время":string)  [unwired: 2 in]
        n143 = Number To Fractional String(number="Т1", precision (6)=w584) -> (F-format string=→"ПОДШ. 1.1":string)  [unwired: 2 in]
        n144 = Number To Fractional String(number="Т2", precision (6)=w584) -> (F-format string=→"ПОДШ. 1.2":string)  [unwired: 2 in]
        n145 = Number To Fractional String(number="Т3", precision (6)=w584) -> (F-format string=→"ПОДШ. 2.1":string)  [unwired: 2 in]
        n146 = Number To Fractional String(number="Т4", precision (6)=w584) -> (F-format string=→"ПОДШ. 2.2":string)  [unwired: 2 in]
        n147 = Number To Fractional String(number="Т5", precision (6)=w584) -> (F-format string=→"ТЕМП РОЛИК":string)  [unwired: 2 in]
        n148 = Number To Fractional String(number="Т6", precision (6)=w584) -> (F-format string=→"ТЕМП КАМЕРА":string)  [unwired: 2 in]
        n149 = call "presure PA.vi"("Volte"="PT3 2") -> ("presure String 2"=→"PT 4":string)  [unwired: 7 in, 3 out]
        n150 = Number To Boolean Array(number="x340") -> (Boolean array=w525:bool[])
        "X340" <- w525
        n151 = Number To Boolean Array(number="x200") -> (Boolean array=→"X200":bool[])
        n152 = Number To Boolean Array(number="x400") -> (Boolean array=→"X400":bool[])
        n153 = Number To Boolean Array(number="y120") -> (Boolean array=→"Y120":bool[])
        n154 = Number To Boolean Array(number="x140") -> (Boolean array=w520:bool[])
        "X140" <- w520
        n155 = Number To Boolean Array(number="x300") -> (Boolean array=→"X300":bool[])
        n156 = Number To Boolean Array(number="x240") -> (Boolean array=→"X240":bool[])
        n157 = Number To Boolean Array(number="x100") -> (Boolean array=w522:bool[])
        "X100" <- w522
        n158 = Number To Boolean Array(number="y60") -> (Boolean array=→"Y60":bool[])
        n159 = local read "V вращ. бараб"() -> (w690:string)
        n160 = local read "V барабаны 2"() -> (→"Частота вращения":dbl)
        n161 = Index Array(array=w729, index #1=2, index #2=5) -> ()  [unwired: 2 out]
        n162 = Number To Fractional String(number="PE3", precision (6)=i16 2) -> (F-format string=→"PE3" →"P камера (bar)":string)  [unwired: 2 in]
        n163 = Number To Fractional String(number="PE1", precision (6)=i16 2) -> (F-format string=→"PE1" →"P плазматрон (bar)":string)  [unwired: 2 in]
        n164 = Number To Fractional String(number="PE2", precision (6)=i16 1) -> (F-format string=→"PE2":string)  [unwired: 2 in]
        n165 = local read "Диаметр заг."() -> (w592:string)
        n166 = Index Array(array=w723, index #1=10, index #2=11, index #3=12) -> (element #1=w717:bool, element #2=w716:bool, element #3=w715:bool)
        n167 = Index Array(array=w658, index #1=18, index #2=29, index #3=30) -> (element #1=w662:bool, element #2=w664:bool, element #3=w665:bool)
        n168 = Index Array(array=w722, index #1=23, index #2=24, index #3=25, index #4=26) -> (element #1=w711:bool, element #2=w710:bool, element #3=w709:bool, element #4=w708:bool)
        n169 = Index Array(array=w803, index #1=16, index #2=18, index #3=19, index #4=20, index #5=21, index #6=24, index #7=25, index #8=28, index #9=29) -> (element #6=→"ролик_прижат":bool, element #7=→"ролик_отжат":bool, element #8=→"УГ_открыт":bool, element #9=→"УГ_закрыт":bool)  [unwired: 5 out]
        n170 = local read "U_ist"() -> (w686:string)
        n171 = To Long Integer(number="Скорость пп 2") -> (32bit integer=w589:i32)
        n172 = To Long Integer(number="Скорость пп") -> (32bit integer=w565:i32)
        n173 = Index Array(array=w784, index #1=1, index #2=6, index #3=7, index #4=27, index #5=14, index #6=13, index #7=21, index #8=22, index #9=23, index #10=24, index #11=25, index #12=19) -> ()  [unwired: 12 out]
        n174 = Index Array(array=w600, index #1=2, index #2=5, index #3=8, index #4=12, index #5=11, index #6=17, index #7=16, index #8=21, index #9=20, index #10=25, index #11=24, index #12=29, index #13=28) -> (element #1=w602:bool, element #2=w606:bool, element #3=w607:bool, element #4=w611:bool, element #5=w612:bool, element #6=w618:bool, element #7=w619:bool, element #8=w626:bool, element #9=w627:bool, element #10=w628:bool, element #11=w629:bool, element #12=w632:bool, element #13=w633:bool)
        n175 = Number To Fractional String(number="M_PLasmatron", precision (6)=i16 1) -> (F-format string=→"voto plasmatron":string)  [unwired: 2 in]
        n176 = Index Array(array=w768, index #1=16, index #2=17, index #3=18, index #4=19, index #5=20, index #6=9, index #7=12, index #8=13, index #9=16, index #10=17, index #11=18, index #12=19, index #13=21, index #14=22, index #15=23, index #16=27, index #17=28, index #18=29) -> (element #1=→"Air":bool, element #2=→"Air 4":bool, element #3=→"давление 1":bool, element #4=→"давление 2":bool)  [unwired: 14 out]
        n177 = Index Array(array=w743, index #1=0, index #2=1, index #3=8, index #4=9, index #5=12, index #6=13, index #7=20, index #8=21, index #9=22, index #10=23, index #11=24, index #12=25, index #13=26, index #14=27, index #15=28, index #16=29, index #17=30, index #18=31) -> (element #7=w742:bool, element #8=w741:bool, element #9=w740:bool, element #10=w739:bool, element #11=w738:bool, element #12=w737:bool, element #13=w736:bool, element #14=w735:bool, element #15=w734:bool, element #16=w733:bool, element #17=w732:bool)  [unwired: 7 out]
        n178 = Index Array(array=w634, index #1=4, index #2=5, index #3=6, index #4=9, index #5=8, index #6=11, index #7=10) -> (element #1=w645:bool, element #2=w646:bool, element #3=w647:bool, element #4=w518:bool, element #5=w517:bool, element #6=w515:bool, element #7=w516:bool)
        n179 = call "Индекс картинки.vi"("ON"=w665, "OFF"=w664) -> ()  [unwired: 9 in, 1 out]
        n180 = Decimal String To Number(string=w686) -> (number=w685:i32)  [unwired: 2 in, 1 out]
        n181 = Decimal String To Number(string=w690) -> (number=w689:i32)  [unwired: 2 in, 1 out]
        n182 = Boolean To (0,1)(Boolean=w717) -> (0, 1=→"EV1":i16)
        n183 = Boolean To (0,1)(Boolean=w716) -> (0, 1=→"EV2":i16)
        n184 = Boolean To (0,1)(Boolean=w711) -> (0, 1=→"CO1":i16)
        n185 = Boolean To (0,1)(Boolean=w710) -> (0, 1=→"CO2":i16)
        n186 = Boolean To (0,1)(Boolean=w709) -> (0, 1=→"CO3":i16)
        n187 = Boolean To (0,1)(Boolean=w708) -> (0, 1=→"P1":i16)
        n188 = Decimal String To Number(string=w592) -> (number=w555:i32)  [unwired: 2 in, 1 out]
        n189 = Boolean To (0,1)(Boolean=w662) -> (0, 1=→"NL2":i16)
        n190 = Number To Decimal String(number=w589) -> (decimal integer string=w591:string)  [unwired: 1 in]
        n191 = Number To Decimal String(number=w565) -> (decimal integer string=w566:string)  [unwired: 1 in]
        n192 = Boolean To (0,1)(Boolean=w715) -> (0, 1=→"EV3.2" →"EV3.3" →"EV3.1":i16)
        n193 = Number To Fractional String(number="V барабаны задание", precision (6)=i16 0) -> (F-format string=→"V задания":string)  [unwired: 2 in]
        n194 = Multiply(x="ЗАДАНИЕ ТОКА", y=1.638) -> (x*y=w569:dbl)
        n195 = local read "Boolean"() -> (w545:bool)
        n196 = call "Индекс картинки.vi"("ON"=w612, "OFF"=w611) -> ("index_image"=→"VP1":u16)  [unwired: 9 in]
        n197 = call "Индекс картинки.vi"("ON"=w619, "OFF"=w618) -> ("index_image"=→"VP2":u16)  [unwired: 9 in]
        n198 = call "Индекс картинки.vi"("ON"=w627, "OFF"=w626) -> ("index_image"=→"VP3":u16)  [unwired: 9 in]
        n199 = call "Индекс картинки.vi"("ON"=w629, "OFF"=w628) -> ("index_image"=→"VP4":u16)  [unwired: 9 in]
        n200 = call "Индекс картинки.vi"("ON"=w633, "OFF"=w632) -> ("index_image"=→"VP5":u16)  [unwired: 9 in]
        n201 = call "Индекс картинки.vi"("ON"=w517, "OFF"=w518) -> ("index_image"=→"PD1":u16)  [unwired: 9 in]
        n202 = call "Индекс картинки.vi"("ON"=w516, "OFF"=w515) -> ("index_image"=→"PD2":u16)  [unwired: 9 in]
        n203 = local write "Скорость ПП 2"(w591) -> ()
        n204 = local write "Скорость ПП"(w566) -> ()
        n205 = Index Array(array=w525, index=4) -> (element=→"Газ":bool)
        n206 = Boolean To (0,1)(Boolean=w602) -> (0, 1=→"NL1":i16)
        n207 = Boolean To (0,1)(Boolean=w607) -> (0, 1=→"NR1":i16)
        n208 = Boolean To (0,1)(Boolean=w606) -> (0, 1=→"NZ1":i16)
        n209 = Boolean To (0,1)(Boolean=w647) -> (0, 1=→"PT3":i16)
        n210 = Boolean To (0,1)(Boolean=w645) -> (0, 1=→"PT1":i16)
        n211 = Boolean To (0,1)(Boolean=w646) -> (0, 1=→"PT2":i16)
        n212 = Index Array(array=w520, index=17) -> (element=→"Распыление":bool)
        n213 = Equal?(x=w555, y=0) -> (x = y?=w558:bool)
        n214 = Greater Or Equal?(x=w685, y=20) -> (x >= y?=w683:bool)
        n215 = Greater Or Equal?(x=w689, y=500) -> (x >= y?=w687:bool)
        n216 = Index Array(array=w522, index=1) -> (element=→"Вакуум":bool)
        n217 = call "Метакон.vi"("Vak_in"="PT4") -> ("Vak_out_txt"=→"PT 4txt":string)  [unwired: 9 in, 1 out]
        n218 = property on="Arhive" class="Bool"() -> ("DisabledEnum"=w543:T7)  [unwired: 2 in, 2 out]
        n219 = And(x=w683, y=w687) -> ()  [unwired: 1 out]
        n220 = To Long Integer(number=w569) -> (32bit integer=w570:i32)
        n221 = Build Array(w742, w741, w740, w739, w738, w737, w736, w735, w734, w733, w732) -> (w529:bool[])
        n222 = Number To Decimal String(number=w570) -> (decimal integer string=w571:string)  [unwired: 1 in]
        n223 = Not Equal?(x=w543, y=T7."Disabled and Grayed Out" ("Disabled")) -> (x != y?=w547:bool)
        n224 = call "4.2 индикар полки.vi"("appended array"=w529) -> ("текущее положение"=→"ИНдикатор положения полки":string)  [unwired: 10 in]
        n225 = Not Equal?(x=w543, y=T7."Enabled") -> (x != y?=w541:bool)
        n226 = case shown="True" w558 {
          tunnel: w555 -> [w806 _]
          tunnel: [w806 210] -> w554
          frame False {
          }
          frame True {
          }
        }
        n227 = And(x=w545, y=w547) -> (x .and. y?=w548:bool)
        n228 = case shown="True" w548 {
          frame False {
          }
          frame True {
            n229 = property on="Arhive" class="Bool"("DisabledEnum"=T7."Disabled and Grayed Out" ("Disabled")) -> ()  [unwired: 2 in, 2 out]
          }
        }
        n230 = Not(x=w545) -> (.not. x?=w544:bool)
        n231 = And(x=w544, y=w541) -> (x .and. y?=w540:bool)
        n232 = local write "задание тока А"(w571) -> ()
        n233 = Number To Decimal String(number="V5014") -> (decimal integer string=w530:string)  [unwired: 1 in]
        n234 = case shown="True" w540 {
          frame False {
          }
          frame True {
            n235 = property on="Arhive" class="Bool"("DisabledEnum"=T7."Enabled" ("Disabled")) -> ()  [unwired: 2 in, 2 out]
          }
        }
        n236 = local write "Пауза допыления"(w530) -> ()
        n237 = Divide(x=210.0, y=w554) -> (x/y=w552:dbl)
        n238 = Multiply(x=9180, y=w552) -> (x*y=w550:dbl)
        n239 = Number To Fractional String(number=w550, precision (6)=i16 0) -> (F-format string=→"max Speed":string)  [unwired: 2 in]
        n240 = Multiply(x="V барабаны", y=w552) -> (x*y=w596:dbl)
        n241 = To Long Integer(number=w596) -> (32bit integer=w557:i32)
        "V барабаны 2" <- w557
        n242 = Number To Fractional String(number=w557, precision (6)=i16 0) -> (F-format string=→"V вращ. бараб":string)  [unwired: 2 in]
        "PT4 2" <- u16 1 ("PT4")
      }
      n243 = while {
        tunnel: w213 -> [w240]
        stop <- FALSE stop-if-true
        w216 = "\t"
        n244 = local read "текущее значение\nзазора (mm)"() -> (w219:string)
        n245 = Wait Until Next ms Multiple(millisecond multiple=u32 1000 ("milliseconds to wait")) -> ()  [unwired: 1 out]
        n246 = local read "ТЕМП КАМЕРА"() -> (w217:string)
        n247 = local read "Скорость ПП 2"() -> (w234:string)
        n248 = local read "V вращ. бараб"() -> (w235:string)
        n249 = local read "ТЕМП РОЛИК"() -> (w223:string)
        n250 = local read "Скорость ПП"() -> (w233:string)
        n251 = Get Date/Time In Seconds() -> (seconds since 1Jan1904=w249:timestamp)
        n252 = local read "ПОДШ. 1.1"() -> (w221:string)
        n253 = local read "ПОДШ. 1.2"() -> (w226:string)
        n254 = local read "ПОДШ. 2.1"() -> (w225:string)
        n255 = local read "ПОДШ. 2.2"() -> (w224:string)
        n256 = Format Date/Time String(seconds (now)=w249) -> (date/time string=w218:string)  [unwired: 2 in]
        n257 = local read "U_ist"() -> (w232:string)
        n258 = local read "PT 1"() -> (w228:string)
        n259 = local read "PT 2"() -> (w227:string)
        n260 = local read "PT 3"() -> (w222:string)
        n261 = local read "PT 4"() -> (w215:string)
        n262 = local read "I_ist"() -> (w220:string)
        n263 = local read "PE1"() -> (w231:string)
        n264 = local read "PE2"() -> (w230:string)
        n265 = local read "PE3"() -> (w229:string)
        n266 = Open/Create/Replace File(file path (use dialog)=w240, error in=errorcluster {"status"=FALSE, "code"=0, "source"=""}) -> (refnum out=w248:refnum<file>, error out=w246:errorcluster)  [unwired: 4 in, 1 out]
        n267 = Concatenate Strings(w218, w216, w219, w216, w220, w216, w235, w216, w234, w216, w233, w216, w232, w216, w231, w216, w230, w216, w229, w216, w228, w216, w227, w216, w222, w216, w221, w216, w226, w216, w225, w216, w224, w216, w223, w216, w217, w216, w215, "\r") -> (w238:string)
        n268 = Set File Position(refnum=w248, from (0:start)=enum16{"start", "end", "current"}."end", error in=w246) -> (refnum out=w245:refnum<file>, error out=w244:errorcluster)  [unwired: 1 in]
        n269 = Write to Text File(file (use dialog)=w245, text=w238, error in=w244) -> (refnum out=w243:refnum<file>, error out=w242:errorcluster)  [unwired: 1 in, 1 out]
        n270 = Close File(refnum=w243, error in=w242) -> (error out=w241:errorcluster)  [unwired: 1 out]
        n271 = Unbundle(w241) -> ()  [unwired: 3 out]
      }
      n272 = while {
        stop <- FALSE stop-if-true
        n273 = event shown="[2] \"Сохранить настройки\": Value Change" {
          selector: _ -> [_ _ _ _ _ _ _ _ _ _ _ _ _ _ _ _ _ _ _ _ _ _ _ _ _ _ _ _ _ _ _]
          dyn-events: _ -> [_ _ _ _ _ _ _ _ _ _ _ _ _ _ _ _ _ _ _ _ _ _ _ _ _ _ _ _ _ _ _]
          timeout: _ -> [_ _ _ _ _ _ _ _ _ _ _ _ _ _ _ _ _ _ _ _ _ _ _ _ _ _ _ _ _ _ _]
          event "Выход": Value Change {
            n274 = event-data() -> ()  [unwired: 1 in, 5 out]
            n275 = Stop(stop? (T)="Выход") -> ()
          }
          event "Arhive": Value Change {
            n276 = event-data() -> ()  [unwired: 1 in, 5 out]
            n277 = call "3.1.форма базы отчетов_UCRI.vi"() -> ()  [unwired: 12 in]
          }
          event "Сохранить настройки": Value Change {
            w299 = i16 0 ("precision (6)")
            n278 = event-data() -> ()  [unwired: 1 in, 5 out]
            n279 = local read "Параметры измерения"() -> (w339:T4)
            n280 = local read "Индикатор камеры 2"() -> (w322:bool)
            n281 = local read "Индикатор камеры"() -> (w349:bool)
            n282 = local read "Уровень бинаризации"() -> (w325:T5)
            n283 = local read "Область измерения"() -> (w348:T3)
            n284 = Unbundle(w339) -> ("Contrast"=w338:i32, "Filter width"=w337:i32, "Steepness"=w336:i32, "Subsampling Ratio"=w335:u32, "Show Search Area"=w334:bool, "Show Search Lines"=w333:bool, "Show Edges Found"=w332:bool, "Show Result"=w331:bool)
            n285 = local read "Рабочий цвет"() -> (w290:u32)
            n286 = local read "Калибровка"() -> (w326:u32)
            n287 = local read "Задержка"() -> (w347:u32)
            n288 = call <vilib>:"Application Directory.vi"() -> ("Application Directory"=w295:path)
            n289 = local read "Фильтр"() -> (w345:i32)
            n290 = Unbundle(w325) -> ("Нижний предел"=w324:sgl, "Верхний предел"=w323:sgl)
            n291 = Boolean To (0,1)(Boolean=w349) -> (0, 1=w346:i16)
            n292 = Boolean To (0,1)(Boolean=w334) -> (0, 1=w330:i16)
            n293 = Boolean To (0,1)(Boolean=w333) -> (0, 1=w329:i16)
            n294 = Boolean To (0,1)(Boolean=w332) -> (0, 1=w328:i16)
            n295 = Boolean To (0,1)(Boolean=w331) -> (0, 1=w327:i16)
            n296 = Boolean To (0,1)(Boolean=w322) -> (0, 1=w302:i16)
            n297 = Unbundle(w348) -> ("Left"=w344:i32, "Top"=w343:i32, "Right"=w342:i32, "Bottom"=w341:i32, "Rotation"=w340:dbl)
            n298 = Path To String(path=w295) -> (string=w294:string)
            n299 = Number To Fractional String(number=w330, precision (6)=w299) -> (F-format string=w309:string)  [unwired: 2 in]
            n300 = Number To Fractional String(number=w329, precision (6)=w299) -> (F-format string=w308:string)  [unwired: 2 in]
            n301 = Number To Fractional String(number=w328, precision (6)=w299) -> (F-format string=w307:string)  [unwired: 2 in]
            n302 = Number To Fractional String(number=w327, precision (6)=w299) -> (F-format string=w306:string)  [unwired: 2 in]
            n303 = Number To Fractional String(number=w347) -> (F-format string=w320:string)  [unwired: 3 in]
            n304 = Number To Fractional String(number=w345) -> (F-format string=w319:string)  [unwired: 3 in]
            n305 = Number To Fractional String(number=w344) -> (F-format string=w318:string)  [unwired: 3 in]
            n306 = Number To Fractional String(number=w343) -> (F-format string=w317:string)  [unwired: 3 in]
            n307 = Number To Fractional String(number=w342) -> (F-format string=w316:string)  [unwired: 3 in]
            n308 = Number To Fractional String(number=w341) -> (F-format string=w315:string)  [unwired: 3 in]
            n309 = Number To Fractional String(number=w340) -> (F-format string=w314:string)  [unwired: 3 in]
            n310 = Number To Fractional String(number=w338) -> (F-format string=w313:string)  [unwired: 3 in]
            n311 = Number To Fractional String(number=w337) -> (F-format string=w312:string)  [unwired: 3 in]
            n312 = Number To Fractional String(number=w336) -> (F-format string=w311:string)  [unwired: 3 in]
            n313 = Number To Fractional String(number=w335) -> (F-format string=w310:string)  [unwired: 3 in]
            n314 = Number To Fractional String(number=w326) -> (F-format string=w305:string)  [unwired: 3 in]
            n315 = Number To Fractional String(number=w324) -> (F-format string=w304:string)  [unwired: 3 in]
            n316 = Number To Fractional String(number=w323) -> (F-format string=w303:string)  [unwired: 3 in]
            n317 = Number To Fractional String(number=w346, precision (6)=i16 0) -> (F-format string=w321:string)  [unwired: 2 in]
            n318 = Number To Fractional String(number=w302, precision (6)=i16 0) -> (F-format string=w301:string)  [unwired: 2 in]
            n319 = Number To Fractional String(number=w290, precision (6)=i16 0) -> (F-format string=w288:string)  [unwired: 2 in]
            n320 = local read "Камера"() -> (w300:T2)
            n321 = Concatenate Strings(w294, "\\set_cam" ("string")) -> (w292:string)
            n322 = Build Array(w300, w321, w320, w319, w318, w317, w316, w315, w314, w313, w312, w311, w310, w309, w308, w307, w306, w305, w304, w303, w301, w288) -> (w296:T2[])
            n323 = String To Path(string=w292) -> (path=w291:path)
            n324 = call-poly <vilib>:"Write To Spreadsheet File.vi"("1D data"=w296, "file path (dialog if empty)"=w291) -> ()  [unwired: 6 in, 1 out]
          }
          event "V задания": Mouse Down {
            (unwired) "" ("ТЕКУЩЕЕ ЗНАЧЕНИЕ")
            n325 = event-data() -> ()  [unwired: 1 in, 7 out]
            n326 = local read "max Speed"() -> (w351:string)
            n327 = local read "V задания"() -> (w352:string)
            n328 = Decimal String To Number(string=w351) -> (number=w350:i32)  [unwired: 2 in, 1 out]
            n329 = call "NUMPAD1_9(ПРОГРАММА).vi"("МИНИМАЛЬНОЕ ЗНАЧЕНИЕ"=-1.0, "МАКСИМАЛЬНОЕ ЗНАЧЕНИЕ"=w350, "ДЛИННА СЛОВА"=i8 5, "ТЕКУЩЕЕ ЗНАЧЕНИЕ"=w352) -> ("НОВОЕ ЗНАЧЕНИЕ"=w354:string)  [unwired: 6 in, 1 out]
            n330 = Fract/Exp String To Number(string=w354) -> (number=w353:dbl)  [unwired: 3 in, 1 out]
            n331 = DataSocket Write(8:errorcluster {"status"=FALSE, "code"=0, "source"=""} ("error in (no error)"), 9:500 ("ms timeout (0)"), 10:w353, 11:"opc://localhost/National Instruments.NIOPCServers/CNL_1.PLC1.PARAM_RASP.SP_S_MOVE" ("connection in")) -> ()  [unwired: 3 out]
          }
          event "Диаметр заг.": Mouse Down {
            n332 = event-data() -> ()  [unwired: 1 in, 7 out]
            n333 = local read "Диаметр заг."() -> (w360:string)
            n334 = call "NUMPAD1_9.vi"("МИНИМАЛЬНОЕ ЗНАЧЕНИЕ"=40.0, "МАКСИМАЛЬНОЕ ЗНАЧЕНИЕ"=90.0, "ДЛИННА СЛОВА"=i8 2, "ТЕКУЩЕЕ ЗНАЧЕНИЕ"=w360) -> ("НОВОЕ ЗНАЧЕНИЕ"=w365:string)  [unwired: 7 in]
            n335 = Fract/Exp String To Number(string=w365) -> (number=w364:dbl)  [unwired: 3 in, 1 out]
            n336 = Multiply(x=w364, y=10.0) -> (x*y=w362:dbl)
            n337 = To Word Integer(number=w362) -> (16bit integer=w361:i16)
            n338 = DataSocket Write(8:errorcluster {"status"=FALSE, "code"=0, "source"=""} ("error in (no error)"), 9:100 ("ms timeout (0)"), 10:w361, 11:"opc://localhost/National Instruments.NIOPCServers/CNL_1.PLC1.PARAM_RASP.D_ZAG") -> (0:w367:errorcluster)  [unwired: 2 out]
            n339 = Unbundle(w367) -> ()  [unwired: 3 out]
          }
          event "ГС -Открыть": Value Change {
            n340 = event-data() -> ()  [unwired: 1 in, 5 out]
            n341 = DataSocket Write(8:errorcluster {"status"=FALSE, "code"=0, "source"=""} ("error in (no error)"), 9:500 ("ms timeout (0)"), 10:TRUE, 11:"" ("connection in")) -> ()  [unwired: 3 out]
          }
          event "ГС - Закрыть": Value Change {
            n342 = event-data() -> ()  [unwired: 1 in, 5 out]
            n343 = DataSocket Write(8:errorcluster {"status"=FALSE, "code"=0, "source"=""} ("error in (no error)"), 9:500 ("ms timeout (0)"), 10:TRUE, 11:"" ("connection in")) -> ()  [unwired: 3 out]
          }
          event "Продол назад": Value Change {
            n344 = event-data() -> ()  [unwired: 1 in, 5 out]
            n345 = DataSocket Write(8:errorcluster {"status"=FALSE, "code"=0, "source"=""} ("error in (no error)"), 9:500 ("ms timeout (0)"), 10:TRUE, 11:"opc://localhost/National Instruments.NIOPCServers/CNL_1.PLC1.Makro.c601" ("connection in")) -> ()  [unwired: 3 out]
          }
          event "ПОДАЧА ЗАГОТОВКИ": Value Change {
            n346 = event-data() -> ()  [unwired: 1 in, 5 out]
            n347 = DataSocket Write(8:errorcluster {"status"=FALSE, "code"=0, "source"=""} ("error in (no error)"), 9:250 ("ms timeout (0)"), 10:TRUE, 11:"opc://localhost/National Instruments.NIOPCServers/DL.DL260.Buttons.Заг-набар" ("connection in")) -> (0:w385:errorcluster)  [unwired: 2 out]
            n348 = Unbundle(w385) -> ()  [unwired: 3 out]
          }
          event "Автораспыление доплавить": Value Change {
            n349 = event-data() -> ()  [unwired: 1 in, 5 out]
          }
          event "Автораспыление начать": Value Change {
            n350 = event-data() -> ()  [unwired: 1 in, 5 out]
            n351 = DataSocket Write(8:errorcluster {"status"=FALSE, "code"=0, "source"=""} ("error in (no error)"), 9:250 ("ms timeout (0)"), 10:TRUE, 11:"opc://localhost/National Instruments.NIOPCServers/DL.DL260.Buttons.расплав-начать" ("connection in")) -> ()  [unwired: 3 out]
          }
          event "ПЛАЗМАТРОН В ИСХОДНОЕ": Value Change {
            n352 = event-data() -> ()  [unwired: 1 in, 5 out]
            n353 = DataSocket Write(8:errorcluster {"status"=FALSE, "code"=0, "source"=""} ("error in (no error)"), 9:500 ("ms timeout (0)"), 10:TRUE, 11:"opc://localhost/National Instruments.NIOPCServers/CNL_1.PLC1.Makro.c600" ("connection in")) -> ()  [unwired: 3 out]
          }
          event "Закончить автораспыление": Value Change {
            n354 = event-data() -> ()  [unwired: 1 in, 5 out]
            n355 = DataSocket Write(8:errorcluster {"status"=FALSE, "code"=0, "source"=""} ("error in (no error)"), 9:250 ("ms timeout (0)"), 10:TRUE, 11:"opc://localhost/National Instruments.NIOPCServers/DL.DL260.Buttons.расплав-закончить" ("connection in")) -> ()  [unwired: 3 out]
          }
          event "Скорость ПП": Mouse Down {
            n356 = event-data() -> ()  [unwired: 1 in, 7 out]
            n357 = call "NUMPAD1_9.vi"("МИНИМАЛЬНОЕ ЗНАЧЕНИЕ"=0.0, "МАКСИМАЛЬНОЕ ЗНАЧЕНИЕ"=601.0, "ДЛИННА СЛОВА"=i8 3, "ТЕКУЩЕЕ ЗНАЧЕНИЕ"="Скорость ПП") -> ("НОВОЕ ЗНАЧЕНИЕ"=w410:string)  [unwired: 7 in]
            n358 = Decimal String To Number(string=w410) -> (number=w402:i32)  [unwired: 2 in, 1 out]
            n359 = To Long Integer(number=w402) -> (32bit integer=w403:i32)
            n360 = DataSocket Write(8:errorcluster {"status"=FALSE, "code"=0, "source"=""} ("error in (no error)"), 9:250 ("ms timeout (0)"), 10:w403, 11:"opc://localhost/National Instruments.NIOPCServers/CNL_1.PLC1.PARAM_RASP.OUT_P_SAG_M" ("connection in")) -> ()  [unwired: 3 out]
            n361 = DataSocket Write(8:errorcluster {"status"=FALSE, "code"=0, "source"=""} ("error in (no error)"), 9:250 ("ms timeout (0)"), 10:w403, 11:"opc://localhost/National Instruments.NIOPCServers/CNL_1.PLC1.PARAM_RASP.4165" ("connection in")) -> ()  [unwired: 3 out]
          }
          event "Скорость ПП 2": Mouse Down {
            n362 = event-data() -> ()  [unwired: 1 in, 7 out]
            n363 = call "NUMPAD1_9.vi"("МИНИМАЛЬНОЕ ЗНАЧЕНИЕ"=0.0, "МАКСИМАЛЬНОЕ ЗНАЧЕНИЕ"=361.0, "ДЛИННА СЛОВА"=i8 3, "ТЕКУЩЕЕ ЗНАЧЕНИЕ"="Скорость ПП 2") -> ("НОВОЕ ЗНАЧЕНИЕ"=w424:string)  [unwired: 7 in]
            n364 = Decimal String To Number(string=w424) -> (number=w416:i32)  [unwired: 2 in, 1 out]
            n365 = To Long Integer(number=w416) -> (32bit integer=w417:i32)
            n366 = DataSocket Write(8:errorcluster {"status"=FALSE, "code"=0, "source"=""} ("error in (no error)"), 9:250 ("ms timeout (0)"), 10:w417, 11:"opc://localhost/National Instruments.NIOPCServers/CNL_1.PLC1.PARAM_RASP.SP_PR_PLAZM" ("connection in")) -> ()  [unwired: 3 out]
            n367 = DataSocket Write(8:errorcluster {"status"=FALSE, "code"=0, "source"=""} ("error in (no error)"), 9:250 ("ms timeout (0)"), 10:w417, 11:"opc://localhost/National Instruments.NIOPCServers/CNL_1.PLC1.PARAM_RASP.4166" ("connection in")) -> ()  [unwired: 3 out]
          }
          event "Пауза допыления": Mouse Down {
            n368 = event-data() -> ()  [unwired: 1 in, 7 out]
            n369 = call "NUMPAD1_9.vi"("МИНИМАЛЬНОЕ ЗНАЧЕНИЕ"=-1.0, "МАКСИМАЛЬНОЕ ЗНАЧЕНИЕ"=10.0, "ДЛИННА СЛОВА"=i8 1, "ТЕКУЩЕЕ ЗНАЧЕНИЕ"="Пауза допыления") -> ("НОВОЕ ЗНАЧЕНИЕ"=w432:string)  [unwired: 7 in]
            n370 = Decimal String To Number(string=w432) -> (number=w431:i32)  [unwired: 2 in, 1 out]
            n371 = DataSocket Write(8:errorcluster {"status"=FALSE, "code"=0, "source"=""} ("error in (no error)"), 9:250 ("ms timeout (0)"), 10:w431, 11:"opc://localhost/National Instruments.NIOPCServers/CNL_1.PLC1.RID.V5014") -> (0:w428:errorcluster)  [unwired: 2 out]
            n372 = Unbundle(w428) -> ()  [unwired: 3 out]
          }
          event "автоматическое включение регулятора": Value Change {
            n373 = event-data() -> ()  [unwired: 1 in, 5 out]
            n374 = DataSocket Write(8:errorcluster {"status"=FALSE, "code"=0, "source"=""} ("error in (no error)"), 9:500 ("ms timeout (0)"), 10:TRUE (".not. x?"), 11:"opc://localhost/National Instruments.NIOPCServers/CNL_1.PLC1.RID.C23") -> (0:w441:errorcluster)  [unwired: 2 out]
            n375 = Unbundle(w441) -> ()  [unwired: 3 out]
          }
          event "МАКСИМАЛЬНАЯ СКОРОСТЬ ПП К": Value Change {
            w443 = "opc://localhost/National Instruments.NIOPCServers/CNL_1.PLC1.PARAM_RASP.SP_PR_PLAZM"  # opc://localhost/National Instruments.NIOPCServers/CNL_1.PLC1.PARAM_RASP.SP_PR_PLAZM
            w447 = "opc://localhost/National Instruments.NIOPCServers/CNL_1.PLC1.PARAM_RASP.SP_PR_ZAG"  # opc://localhost/National Instruments.NIOPCServers/CNL_1.PLC1.PARAM_RASP.SP_PR_ZAG
            n376 = event-data() -> ()  [unwired: 1 in, 5 out]
            n377 = DataSocket Write(8:errorcluster {"status"=FALSE, "code"=0, "source"=""} ("error in (no error)"), 10:600, 11:w447) -> ()  [unwired: 1 in, 3 out]
            n378 = DataSocket Write(8:errorcluster {"status"=FALSE, "code"=0, "source"=""} ("error in (no error)"), 10:360, 11:w443) -> ()  [unwired: 1 in, 3 out]
          }
          event "задание тока А": Mouse Down {
            n379 = event-data() -> ()  [unwired: 1 in, 7 out]
            n380 = call "NUMPAD1_9.vi"("МИНИМАЛЬНОЕ ЗНАЧЕНИЕ"=0.0, "МАКСИМАЛЬНОЕ ЗНАЧЕНИЕ"=2500.0, "ДЛИННА СЛОВА"=i8 4, "ТЕКУЩЕЕ ЗНАЧЕНИЕ"="задание тока А") -> ("НОВОЕ ЗНАЧЕНИЕ"=w457:string)  [unwired: 7 in]
            n381 = Decimal String To Number(string=w457) -> (number=w456:i32)  [unwired: 2 in, 1 out]
            n382 = Multiply(x=w456, y=1.638) -> (x*y=w454:dbl)
            n383 = To Long Integer(number=w454) -> (32bit integer=w453:i32)
            n384 = DataSocket Write(8:errorcluster {"status"=FALSE, "code"=0, "source"=""} ("error in (no error)"), 9:250 ("ms timeout (0)"), 10:w453, 11:"opc://localhost/National Instruments.NIOPCServers/DL.DL260.Vmem.ист-задание" ("connection in")) -> ()  [unwired: 3 out]
          }
          event "Улавливатель закрыть": Value Change {
            n385 = event-data() -> ()  [unwired: 1 in, 5 out]
          }
          event "Улавливатель открыть": Value Change {
            n386 = event-data() -> ()  [unwired: 1 in, 5 out]
          }
          event "Ролик прижать": Value Change {
            n387 = event-data() -> ()  [unwired: 1 in, 5 out]
            n388 = DataSocket Write(8:errorcluster {"status"=FALSE, "code"=0, "source"=""} ("error in (no error)"), 9:500 ("ms timeout (0)"), 10:TRUE, 11:"opc://localhost/National Instruments.NIOPCServers/DL.DL260.Buttons.Рол-прижать" ("connection in")) -> ()  [unwired: 3 out]
          }
          event "Ролик отжать": Value Change {
            n389 = event-data() -> ()  [unwired: 1 in, 5 out]
            n390 = DataSocket Write(8:errorcluster {"status"=FALSE, "code"=0, "source"=""} ("error in (no error)"), 9:500 ("ms timeout (0)"), 10:TRUE, 11:"opc://localhost/National Instruments.NIOPCServers/DL.DL260.Buttons.Рол-отжать" ("connection in")) -> ()  [unwired: 3 out]
          }
          event "откачать рабочий вакуум": Value Change {
            n391 = event-data() -> ()  [unwired: 1 in, 5 out]
            n392 = property on="откачать рабочий вакуум" class="Bool"() -> ("BoolText.Text"=w474:string)  [unwired: 2 in, 2 out]
            n393 = call "Диалог_на_Макро.vi"("СОСТОЯНИЕ"="mac 2", "String"=w474) -> ("ВЫХОД"=w470:bool)  [unwired: 8 in, 1 out]
            n394 = DataSocket Write(9:500 ("ms timeout (0)"), 10:w470, 11:"opc://localhost/National Instruments.NIOPCServers/CNL_1.PLC1.Makro.c200" ("connection in")) -> (0:w473:errorcluster)  [unwired: 1 in, 2 out]
            n395 = Unbundle(w473) -> ()  [unwired: 3 out]
          }
          event "forvacuum": Value Change {
            n396 = event-data() -> ()  [unwired: 1 in, 5 out]
            n397 = property on="forvacuum" class="Bool"() -> ("BoolText.Text"=w475:string)  [unwired: 2 in, 2 out]
            n398 = call "Диалог_на_Макро.vi"("СОСТОЯНИЕ"="forvakuum led", "String"=w475) -> ("ВЫХОД"=w480:bool)  [unwired: 8 in, 1 out]
            n399 = DataSocket Write(9:500 ("ms timeout (0)"), 10:w480, 11:"opc://localhost/National Instruments.NIOPCServers/CNL_1.PLC1.Makro.c251" ("connection in")) -> (0:w477:errorcluster)  [unwired: 1 in, 2 out]
            n400 = Unbundle(w477) -> ()  [unwired: 3 out]
          }
          event "ND HEAT BUT": Value Change {
            n401 = event-data() -> ()  [unwired: 1 in, 5 out]
            n402 = property on="ND HEAT BUT" class="Bool"() -> ("BoolText.Text"=w481:string)  [unwired: 2 in, 2 out]
            n403 = call "Диалог_на_Макро.vi"("СОСТОЯНИЕ"="ND HEAT LED", "String"=w481) -> ("ВЫХОД"=w486:bool)  [unwired: 8 in, 1 out]
            n404 = DataSocket Write(9:500 ("ms timeout (0)"), 10:w486, 11:"opc://localhost/National Instruments.NIOPCServers/CNL_1.PLC1.Makro.c250" ("connection in")) -> (0:w483:errorcluster)  [unwired: 1 in, 2 out]
            n405 = Unbundle(w483) -> ()  [unwired: 3 out]
          }
          event "откачка стоп": Value Change {
            n406 = event-data() -> ()  [unwired: 1 in, 5 out]
            n407 = property on="откачка стоп" class="Bool"() -> ("BoolText.Text"=w487:string)  [unwired: 2 in, 2 out]
            n408 = call "Диалог_на_Макро.vi"("СОСТОЯНИЕ"="mac3", "String"=w487) -> ("ВЫХОД"=w489:bool)  [unwired: 8 in, 1 out]
            n409 = DataSocket Write(9:500 ("ms timeout (0)"), 10:w489, 11:"opc://localhost/National Instruments.NIOPCServers/CNL_1.PLC1.Makro.c201" ("connection in")) -> (0:w492:errorcluster)  [unwired: 1 in, 2 out]
            n410 = Unbundle(w492) -> ()  [unwired: 3 out]
          }
          event "напустить газ в камеру": Value Change {
            n411 = event-data() -> ()  [unwired: 1 in, 5 out]
            n412 = property on="напустить газ в камеру" class="Bool"() -> ("BoolText.Text"=w498:string)  [unwired: 2 in, 2 out]
            n413 = call "Диалог_на_Макро.vi"("СОСТОЯНИЕ"="mac 4", "String"=w498) -> ("ВЫХОД"=w493:bool)  [unwired: 8 in, 1 out]
            n414 = DataSocket Write(9:500 ("ms timeout (0)"), 10:w493, 11:"opc://localhost/National Instruments.NIOPCServers/CNL_1.PLC1.Makro.napusk" ("connection in")) -> (0:w496:errorcluster)  [unwired: 1 in, 2 out]
            n415 = Unbundle(w496) -> ()  [unwired: 3 out]
          }
          event "напустить гелий в ресивер": Value Change {
            n416 = event-data() -> ()  [unwired: 1 in, 5 out]
            n417 = property on="напустить гелий в ресивер" class="Bool"() -> ("BoolText.Text"=w499:string)  [unwired: 2 in, 2 out]
            n418 = call "Диалог_на_Макро.vi"("СОСТОЯНИЕ"="mac5", "String"=w499) -> ("ВЫХОД"=w502:bool)  [unwired: 8 in, 1 out]
            n419 = DataSocket Write(9:500 ("ms timeout (0)"), 10:w502, 11:"opc://localhost/National Instruments.NIOPCServers/CNL_1.PLC1.Makro.C610") -> (0:w504:errorcluster)  [unwired: 1 in, 2 out]
            n420 = Unbundle(w504) -> ()  [unwired: 3 out]
          }
          event "напустить аргон в ресивер": Value Change {
            n421 = event-data() -> ()  [unwired: 1 in, 5 out]
            n422 = property on="напустить аргон в ресивер" class="Bool"() -> ("BoolText.Text"=w505:string)  [unwired: 2 in, 2 out]
            n423 = call "Диалог_на_Макро.vi"("СОСТОЯНИЕ"="mac6", "String"=w505) -> ("ВЫХОД"=w508:bool)  [unwired: 8 in, 1 out]
            n424 = DataSocket Write(9:500 ("ms timeout (0)"), 10:w508, 11:"opc://localhost/National Instruments.NIOPCServers/CNL_1.PLC1.Makro.C611") -> (0:w510:errorcluster)  [unwired: 1 in, 2 out]
            n425 = Unbundle(w510) -> ()  [unwired: 3 out]
          }
          event "ЗУ-вверх": Value Change {
            n426 = event-data() -> ()  [unwired: 1 in, 5 out]
            n427 = DataSocket Write(8:errorcluster {"status"=FALSE, "code"=0, "source"=""} ("error in (no error)"), 9:500 ("ms timeout (0)"), 10:TRUE, 11:"opc://localhost/National Instruments.NIOPCServers/CNL_1.PLC1.Makro.s226" ("connection in")) -> ()  [unwired: 3 out]
          }
        }
        n428 = Wait Until Next ms Multiple(millisecond multiple=u32 500) -> ()  [unwired: 1 out]
      }
      n429 = while {
        stop <- FALSE stop-if-true
        n430 = Get Date/Time In Seconds() -> (seconds since 1Jan1904=w256:timestamp)
        n431 = Wait (ms)(milliseconds to wait=u32 500) -> ()  [unwired: 1 out]
        n432 = Format Date/Time String(seconds (now)=w256) -> (date/time string=w250:string)  [unwired: 2 in]
        n433 = Greater?(x="Ошибка 2", y=i16 0) -> (0:w252:bool)
        n434 = case shown="True" w252 {
          tunnel: "Ошибка 2" -> [_ w259]
          tunnel: w250 -> [_ w267]
          frame False {
          }
          frame True {
            w261 = "\r"
            w269 = "\t"
            n435 = call "4.1. описание ошибки.vi"("Numeric"=w259) -> ("Сообщение"=w257:string, "Механизм"=w258:string)  [unwired: 8 in, 1 out]
            n436 = local write "Ошибка 2"(i16 0 ("Ошибка 2")) -> ()
            n437 = Number To Decimal String(number=w259) -> (decimal integer string=w265:string)  [unwired: 1 in]
            n438 = call "путь для общего отчета.vi"() -> ("path_out 2"=w270:string)  [unwired: 11 in]
            n439 = Concatenate Strings(w267, w269, w265, w269, w258, "   " ("string"), w257, "\n") -> (w271:string)
            n440 = Concatenate Strings("Data: " ("string"), w267, w261, "Numer: " ("string"), w265, w261, w258, w261, w257) -> (w264:string)
            n441 = Concatenate Strings(w270, "errors.txt") -> (w282:string)
            n442 = call "2.6. форма ошибки.vi"("Описание ошибки"=w264) -> ()  [unwired: 11 in]
            n443 = String To Path(string=w282) -> (path=w284:path)
            n444 = Open/Create/Replace File(file path (use dialog)=w284, error in=errorcluster {"status"=FALSE, "code"=0, "source"=""}, operation (0:open)=T6."open or create") -> (refnum out=w277:refnum<file>, error out=w279:errorcluster)  [unwired: 3 in, 1 out]
            n445 = Set File Position(refnum=w277, from (0:start)=enum16{"start", "end", "current"}."end", error in=w279) -> (refnum out=w275:refnum<file>, error out=w276:errorcluster)  [unwired: 1 in]
            n446 = Write to Text File(file (use dialog)=w275, text=w271, error in=w276) -> (refnum out=w274:refnum<file>, error out=w273:errorcluster)  [unwired: 1 in, 1 out]
            n447 = Close File(refnum=w274, error in=w273) -> (error out=w272:errorcluster)  [unwired: 1 out]
            n448 = Unbundle(w272) -> ()  [unwired: 3 out]
          }
        }
      }
    }
  }
  n449 = while {
    stop <- FALSE stop-if-true
    n450 = flat-sequence {
      tunnel: [w903] -> w810
      frame #0 {
        n451 = call <vilib>:"Application Directory.vi"() -> ("Application Directory"=w817:path)
        n452 = Path To String(path=w817) -> (string=w816:string)
        n453 = Concatenate Strings(w816, "\\set_cam" ("string")) -> (w814:string)
        n454 = String To Path(string=w814) -> (path=w811:path)
        n455 = Get File Size(file=w811) -> (0:w813:errorcluster)  [unwired: 1 in, 2 out]
        n456 = Unbundle By Name(w813) -> ("status"=w812:bool)
        n457 = case shown="False" w812 {
          tunnel: w811 -> [w890 _]
          frame False {
            n458 = call-poly <vilib>:"Read From Spreadsheet File.vi"("file path (dialog if empty)"=w890) -> ("first row"=w889:string[])  [unwired: 6 in, 4 out]
            n459 = Index Array(array=w889, index #1=0 ("index"), index #2=2 ("index"), index #3=3 ("index"), index #4=4 ("index"), index #5=5 ("index"), index #6=6 ("index"), index #7=7 ("index"), index #8=8 ("index"), index #9=9 ("index"), index #10=10 ("index"), index #11=11 ("index"), index #12=12 ("index"), index #13=13 ("index"), index #14=14 ("index"), index #15=15 ("index"), index #16=16 ("index"), index #17=17 ("index"), index #18=18 ("index"), index #19=19 ("index"), index #20=20 ("index"), index #21=21 ("index")) -> (element #1=w887:string, element #2=w885:string, element #3=w882:string, element #4=w874:string, element #5=w872:string, element #6=w870:string, element #7=w868:string, element #8=w866:string, element #9=w857:string, element #10=w855:string, element #11=w853:string, element #12=w851:string, element #13=w849:string, element #14=w847:string, element #15=w845:string, element #16=w843:string, element #17=w833:string, element #18=w828:string, element #19=w826:string, element #20=w822:string, element #21=w818:string)
            n460 = local write "Камера"(w887) -> ()
            n461 = Decimal String To Number(string=w885) -> (number=w884:i32)  [unwired: 2 in, 1 out]
            n462 = Decimal String To Number(string=w882) -> (number=w881:i32)  [unwired: 2 in, 1 out]
            n463 = Decimal String To Number(string=w874) -> (number=w879:i32)  [unwired: 2 in, 1 out]
            n464 = Decimal String To Number(string=w872) -> (number=w878:i32)  [unwired: 2 in, 1 out]
            n465 = Decimal String To Number(string=w870) -> (number=w877:i32)  [unwired: 2 in, 1 out]
            n466 = Decimal String To Number(string=w868) -> (number=w876:i32)  [unwired: 2 in, 1 out]
            n467 = Fract/Exp String To Number(string=w866) -> (number=w865:dbl)  [unwired: 3 in, 1 out]
            n468 = Decimal String To Number(string=w857) -> (number=w863:i32)  [unwired: 2 in, 1 out]
            n469 = Decimal String To Number(string=w855) -> (number=w862:i32)  [unwired: 2 in, 1 out]
            n470 = Decimal String To Number(string=w853) -> (number=w861:i32)  [unwired: 2 in, 1 out]
            n471 = Decimal String To Number(string=w851) -> (number=w860:i32)  [unwired: 2 in, 1 out]
            n472 = Decimal String To Number(string=w849) -> (number=w842:i32)  [unwired: 2 in, 1 out]
            n473 = Decimal String To Number(string=w847) -> (number=w840:i32)  [unwired: 2 in, 1 out]
            n474 = Decimal String To Number(string=w845) -> (number=w838:i32)  [unwired: 2 in, 1 out]
            n475 = Decimal String To Number(string=w843) -> (number=w836:i32)  [unwired: 2 in, 1 out]
            n476 = Decimal String To Number(string=w833) -> (number=w832:i32)  [unwired: 2 in, 1 out]
            n477 = Decimal String To Number(string=w828) -> (number=w827:i32)  [unwired: 2 in, 1 out]
            n478 = Decimal String To Number(string=w826) -> (number=w825:i32)  [unwired: 2 in, 1 out]
            n479 = Decimal String To Number(string=w822) -> (number=w824:i32)  [unwired: 2 in, 1 out]
            n480 = Decimal String To Number(string=w818) -> (number=w820:i32)  [unwired: 2 in, 1 out]
            n481 = To Unsigned Long Integer(number=w860) -> (unsigned 32bit integer=w859:u32)
            n482 = local write "Задержка"(w884) -> ()
            n483 = local write "Фильтр"(w881) -> ()
            n484 = Bundle(w879, w878, w877, w876, w865) -> (w880:cluster{i32, i32, i32, i32, dbl})  [unwired: 1 in]
            n485 = call "конвертюга.vi"("Numeric"=w842) -> ("Boolean"=w841:bool)  [unwired: 10 in]
            n486 = call "конвертюга.vi"("Numeric"=w840) -> ("Boolean"=w839:bool)  [unwired: 10 in]
            n487 = call "конвертюга.vi"("Numeric"=w838) -> ("Boolean"=w837:bool)  [unwired: 10 in]
            n488 = call "конвертюга.vi"("Numeric"=w836) -> ("Boolean"=w835:bool)  [unwired: 10 in]
            n489 = local write "Калибровка"(w832) -> ()
            n490 = Bundle(w827, w825) -> (w831:cluster{i32, i32})  [unwired: 1 in]
            n491 = call "конвертюга.vi"("Numeric"=w824) -> ("Boolean"=w823:bool)  [unwired: 10 in]
            n492 = local write "Рабочий цвет"(w820) -> ()
            n493 = local write "Область измерения"(w880) -> ()
            n494 = local write "Уровень бинаризации"(w831) -> ()
            n495 = local write "Blank Button"(w823) -> ()
            n496 = Bundle(w863, w862, w861, w859, "Boolean"=w841, "Boolean"=w839, "Boolean"=w837, "Boolean"=w835) -> (w864:T8)  [unwired: 1 in]
            n497 = local write "Параметры измерения"(w864) -> ()
          }
          frame True {
          }
        }
      }
      frame #1 {
        n498 = case shown="True" FALSE {
          frame False {
          }
          frame True {
            n499 = while {
              stop <- "Play Button" stop-if-true
              "Индикатор камеры" <- FALSE ("Индикатор камеры")
            }
          }
        }
      }
      frame #2 {
        w895 = T9 4 items=["Grayscale (U8)", "Grayscale (I16)", "Grayscale (SGL)", "Complex (CSG)", "RGB (U32)", "HSL (U32)", "RGB (U64)", "Grayscale (U16)"] ("Image Type")
        w900 = T9 4 items=["Grayscale (U8)", "Grayscale (I16)", "Grayscale (SGL)", "Complex (CSG)", "RGB (U32)", "HSL (U32)", "RGB (U64)", "Grayscale (U16)"] ("Image Type")
        n500 = call <vilib>:"IMAQdx Open Camera.vi"("Session In"="Камера") -> ("Session Out"=w902:T2)  [unwired: 9 in, 1 out]
        n501 = call <vilib>:"IMAQdx Configure Grab.vi"("Session In"=w902) -> ("Session Out"=w898:T2)  [unwired: 9 in, 1 out]
        n502 = call "IMAQ Create"("Image Name"="capture", "Image Type"=w900) -> ("New Image"=w897:T1)  [unwired: 3 in, 1 out]
        n503 = call "IMAQ Create"("Image Name"="capture2", "Image Type"=w895) -> ("New Image"=w894:T1)  [unwired: 3 in, 1 out]
        n504 = while {
          tunnel: [w917] -> w903
          tunnel: w898 -> [w907]
          tunnel: w897 -> [w906]
          tunnel: w894 -> [w904]
          stop <- "Media Stop Button" stop-if-true
          n505 = flat-sequence {
            tunnel: [w921] -> w916
            tunnel: [w918] -> w914
            tunnel: w907 -> [w920]
            tunnel: w906 -> [w919]
            tunnel: [w918] -> w905
            tunnel: w916 -> [w932]
            tunnel: [w932] -> w915
            tunnel: w914 -> [w931]
            tunnel: [w931] -> w913
            tunnel: w905 -> [w930]
            tunnel: w904 -> [w926]
            tunnel: w915 -> [w952]
            tunnel: w913 -> [w951]
            tunnel: [w952] -> w912
            tunnel: [w950] -> w909
            tunnel: w912 -> [w974]
            tunnel: [w974] -> w911
            tunnel: [w973] -> w910
            tunnel: w909 -> [w973]
            tunnel: [w976] -> w917
            tunnel: w911 -> [w976]
            tunnel: w910 -> [w975]
            frame #0 {
              n506 = local write "Индикатор камеры"(TRUE ("Индикатор камеры")) -> ()
              n507 = call <vilib>:"IMAQdx Grab.vi"("Image In"=w919, "Session In"=w920) -> ("Image Out"=w918:T1, "Session Out"=w921:T2)  [unwired: 6 in, 2 out]
            }
            frame #1 {
              w925 = u32 1 items=["Horizontal", "Vertical", "Central", "1st Diagonal", "2nd Diagonal"] ("Type of Symmetry")
              n508 = call "IMAQ Copy"("Image Dst"=w926, "Image Src"=w930) -> ("Image Dst Out"=w928:T1)  [unwired: 4 in, 1 out]
              n509 = call "IMAQ Symmetry"("Type of Symmetry"=w925, "Image Dst"=w926, "Image Src"=w928) -> ("Image Dst Out"=w927:T1)  [unwired: 2 in, 1 out]
              n510 = call-poly "IMAQ Write File 2"("error in (no error)"=errorcluster {"status"=FALSE, "code"=0, "source"=""}, "File Path"=path "D:/image", "Image"=w927) -> ("error out"=w923:errorcluster)  [unwired: 7 in, 1 out]
              n511 = Unbundle(w923) -> ()  [unwired: 3 out]
            }
            frame #2 {
              (unwired) 7 items=["Red", "Green", "Blue", "Hue", "Saturation", "Luminance", "Value", "Intensity"] ("Color Plane")
              (unwired) u32 8487297 ("Color Box")
              (unwired) 612
              n512 = Wait (ms)(milliseconds to wait="Задержка") -> ()  [unwired: 1 out]
              n513 = Increment(x="Numeric") -> (x+1=w953:i16)
              n514 = local write "Numeric"(w953) -> ()
              n515 = call "IMAQ Subtract"("Image Src A"=w951, "Constant"="Калибровка") -> ("Image Dst Out"=w961:T1)  [unwired: 5 in, 1 out]
              n516 = call "IMAQ ExtractSingleColorPlane"("Color Plane"="Фильтр", "Image Src"=w961) -> ("Image Dst Out"=w940:T1)  [unwired: 8 in, 1 out]
              n517 = case shown="True" "Blank Button" {
                tunnel: w940 -> [w968 w972]
                tunnel: [w968 w971] -> w947
                frame False {
                }
                frame True {
                  (unwired) cluster{"Lower value":sgl, "Upper value":sgl} {"Lower value"=124.0, "Upper value"=255.0} ("Range")
                  (unwired) u32 16448250 ("Color Box 2")
                  n518 = call "IMAQ Threshold"("Replace Value"="Рабочий цвет", "Range"="Уровень бинаризации", "Image Src"=w972) -> ("Image Dst Out"=w971:T1)  [unwired: 3 in, 5 out]
                }
              }
              n519 = Unbundle("Область измерения") -> ("Top"=w937:i32, "Bottom"=w936:i32)  [unwired: 3 out]
              n520 = Greater?(x=w937, y=w936) -> (0:w939:bool)
              n521 = case shown="False" w939 {
                tunnel: [w965 w967] -> w938
                tunnel: w937 -> [w964 w967]
                tunnel: w936 -> [w965 w966]
                tunnel: [w964 w966] -> w935
                frame False {
                }
                frame True {
                }
              }
              n522 = Subtract(x=w938, y=w935) -> (x-y=w945:i32)
              n523 = Multiply(x="D, заготовки", y=i16 10) -> (x*y=w942:i16)
              n524 = Divide(x=w942, y=w945) -> (x/y=w941:dbl)
              "x/y" <- w941
              n525 = call "IMAQ Clamp Horizontal Max"("Settings"="Параметры измерения", "Rectangle"="Область измерения", "Image"=w947) -> ("Distance"=w959:sgl, "Image Out"=w950:T1)  [unwired: 4 in, 3 out]
              "Distance зазор" <- w959
              n526 = Multiply(x=w959, y=w941) -> (x*y=w957:dbl)
              "x*y" <- w957
              n527 = Divide(x=w957, y=10.0) -> (x/y=w955:dbl)
              n528 = To Word Integer(number=w955) -> (16bit integer=→"16bit integer":i16)
              n529 = Divide(x=800, y=574) -> ()  [unwired: 1 out]
              "Индикатор камеры 2" <- "Blank Button"
            }
            frame #3 {
            }
            frame #4 {
              "индикация видео" <- w975
            }
          }
        }
      }
    }
    n530 = Wait Until Next ms Multiple(millisecond multiple=u32 10) -> ()  [unwired: 1 out]
    n531 = call <vilib>:"IMAQdx Close Camera.vi"("Session In"=w810) -> ()  [unwired: 10 in, 1 out]
  }
